vi "eyecat MAX v02.vi"() -> ()   [LabVIEW 2014]
doc: "This VI is an upgrade from the WIN 1_v4 that implements the ageing subrutine"
uses:
  Buttons/String output.ctl
  <vilib>/Utility/miscctls.llb/LVRowAndColumnTypeDef.ctl
  Buttons/Numeric control.ctl
  Buttons/String input.ctl
  Buttons/Numeric indicator.ctl
  Controls Win/Control 3.ctl
  <vilib>/Platform/TimedLoop/XDataNode/nitl_modes.ctl
  <vilib>/Platform/TimedLoop/XDataNode/timing_clust.ctl
  <vilib>/Platform/TimedLoop/XDataNode/wakeup.ctl
  <vilib>/Utility/file.llb/Write To Spreadsheet File (string).vi
  <vilib>/Utility/file.llb/Read From Spreadsheet File (string).vi
  <vilib>/regexp/Match Regular Expression.xnode
  <vilib>/Platform/TimedLoop/XDataNode/XDataNode.xnode
  <vilib>/Platform/TimedLoop/XDataNode/XDNodeRunTimeDep.lvlib
panel:
  out "Furnace temp 2":dbl
  out "output cluster":T2
  out "Full system?":bool
  out "Log interval (seconds)":T1
  in  "Flow rate Age":dbl
  in  "Inlet temp Age":dbl
  out "Stopped?":bool
  in  "Stop Cmd":T1
  out "Connected?":bool
  out "Error":dbl
  out "Iteration Duration":i64
  out "Finished Late? [i-1]":bool
  in  "stop TCP":bool
  in  "SO2 ppm":dbl
  out "Furnace temp 1":dbl
  out "stop 2":bool
  in  "Enum 1":i16=1
  in  "Acknowledge":bool
  out "Test number":u16
  out "Flag1":bool=TRUE
  out "EditPos Subc":T3
  out "Flag 2":bool=TRUE
  in  "Tab Control":T4(tab)
  out "Doors Unlocked":bool
  in  "Temperature Limit (°C)":T1=800.0 min=0.0 max=1200.0 step=1.0
  in  "Log Test Button":bool
  in  "File Name":T5
  in  "File Path":path=path "C:/DATA LOG"
  out "Fail":bool
  out "Pass":bool
  in  "Select Test Type":T6(radio)
  out "Standby":bool
  out "Doors Open":bool
  out "Extractor Fan On":bool
  out "Test In Progress":bool
  out "Cool Down":bool
  out "System Alarm":bool
  in  "Execute Leak Test Button":bool
  in  "Stop Test Button":bool
  in  "Start Test Button":bool
  in  "Advanced settings":bool
  in  "Inlet Temperature (°C)":T1=400.0 min=350.0 max=1000.0 step=1.0
  in  "Inlet LAMBDA Rich":T1=0.9 min=0.85 max=0.96 step=0.001
  in  "Inlet LAMBDA Lean":T1=1.2 min=1.02 max=3.0 step=0.001
  in  "Test Stop temperature (°C)":T1=300.0 min=100.0 max=1000.0 step=1.0
  in  "Test Start Temperature (°C)":T1=125.0 min=0.0 max=500.0 step=1.0
  in  "Furnace Ramp Rate (°C/min)":T1=15.0 min=1.0 max=50.0 step=0.1
  in  "NO:CO Ratio":T1=1.1 min=1.0 max=5.0 step=0.1
  in  "Inlet O2 (%)":T1=0.5 min=0.0 max=14.0 step=0.01
  in  "Inlet LAMBDA":T1=1.0 min=0.6 max=3.0 step=0.001
  out "Space Velocity (h-1)":T7
  out "Vol Flow @ STP (l/min)":T7
  in  "Test Flow Rate(g/s)":T1 min=0.0 max=100.0 step=0.01
  out "Sample Volume (litres)":T7
  in  "Number of Samples":T1=1.0 min=1.0 max=6.0 step=1.0
  in  "Sample Diameter (mm)":T1
  out "CO Theory (%)":T7 format="%#_3g"
  out "CO Theory (%)":T7 format="%#_3g"
  out "HC Theory (%)":T7
  in  "Sample Length (mm)":T1 min=0.0 step=0.5
  in  "NO ppm SW":dbl=500.0 caption="NO (ppm)" min=0.0 max=500.0 step=1.0
  in  "NO ppm Loff":T1 caption="NO ppm"
  in  "Delete sCycle":bool
  in  "Load sCycle":bool
  in  "Save sCycle":bool
  in  "Clear subcycle":bool
  in  "Clear Cycle Pattern":bool
  in  "Save Cycle":bool
  in  "Load Cycle":bool
  in  "Delete Cycle":bool
  out "Test Compiled":bool
  in  "Compile Test Button":bool
  in  "Sub-Cycle List":i32(listbox)=1
  in  "Cycle List":i32(listbox)=2
  out "Total Test Duration (hrs)":T8
  in  "Ageing Gas":enum32{"Radio Selection 1", "Radio Selection 2"}(radio)
  in  "Sub-Cycle Pattern":string[][](table) caption="Subcycle pattern"
  in  "Total Number of Cycles":T1=1.0 min=1.0 max=10000.0 step=1.0
  in  "Cycle Pattern":string[][](table)
  in  "Sub-Cycle Name":T5
  in  "Cycle Name":T5
  out "Heat Exchanger Temperatures (°C)":dynamicdata(graph)
  out "Flow Rate (g/s)":dynamicdata(graph)
  out "Sample Temperatures (°C)":dynamicdata(graph)
  out "System Temperatures (°C)":dynamicdata(graph)
  out "HC Concentration (ppm)":dynamicdata(graph)
  out "Lambda":dynamicdata(graph)
  out "M584L Upstream & Downstream":dynamicdata(graph)
  out "NO Concentration (ppm)":dynamicdata(graph)
  in  "Purge System":bool
  in  "Alarm ack":bool
  in  "Clear log":bool
  out "Table":string[][](table)
  out "Soft Alarm":bool
  out "Hard Alarm":bool
  # "Test Type"
  # "Test Commands"
  # "System Indicators"
  # "Leak Test"
  # "Catalyst Specification"
  # "Lightoff Settings"
  # "Furnace Lightoff Settings"
  # "Sweep Settings"
  # "CO/HC Lightoff Settings"
  # "0.96 < lambda < 0.85"
  # "1.02< lambda < 1.6"
  # "350 < Tinlet < 1000"
  # "NO Lightoff Settings"
  # "Flow Specification"
  # "Cycle Compiled"
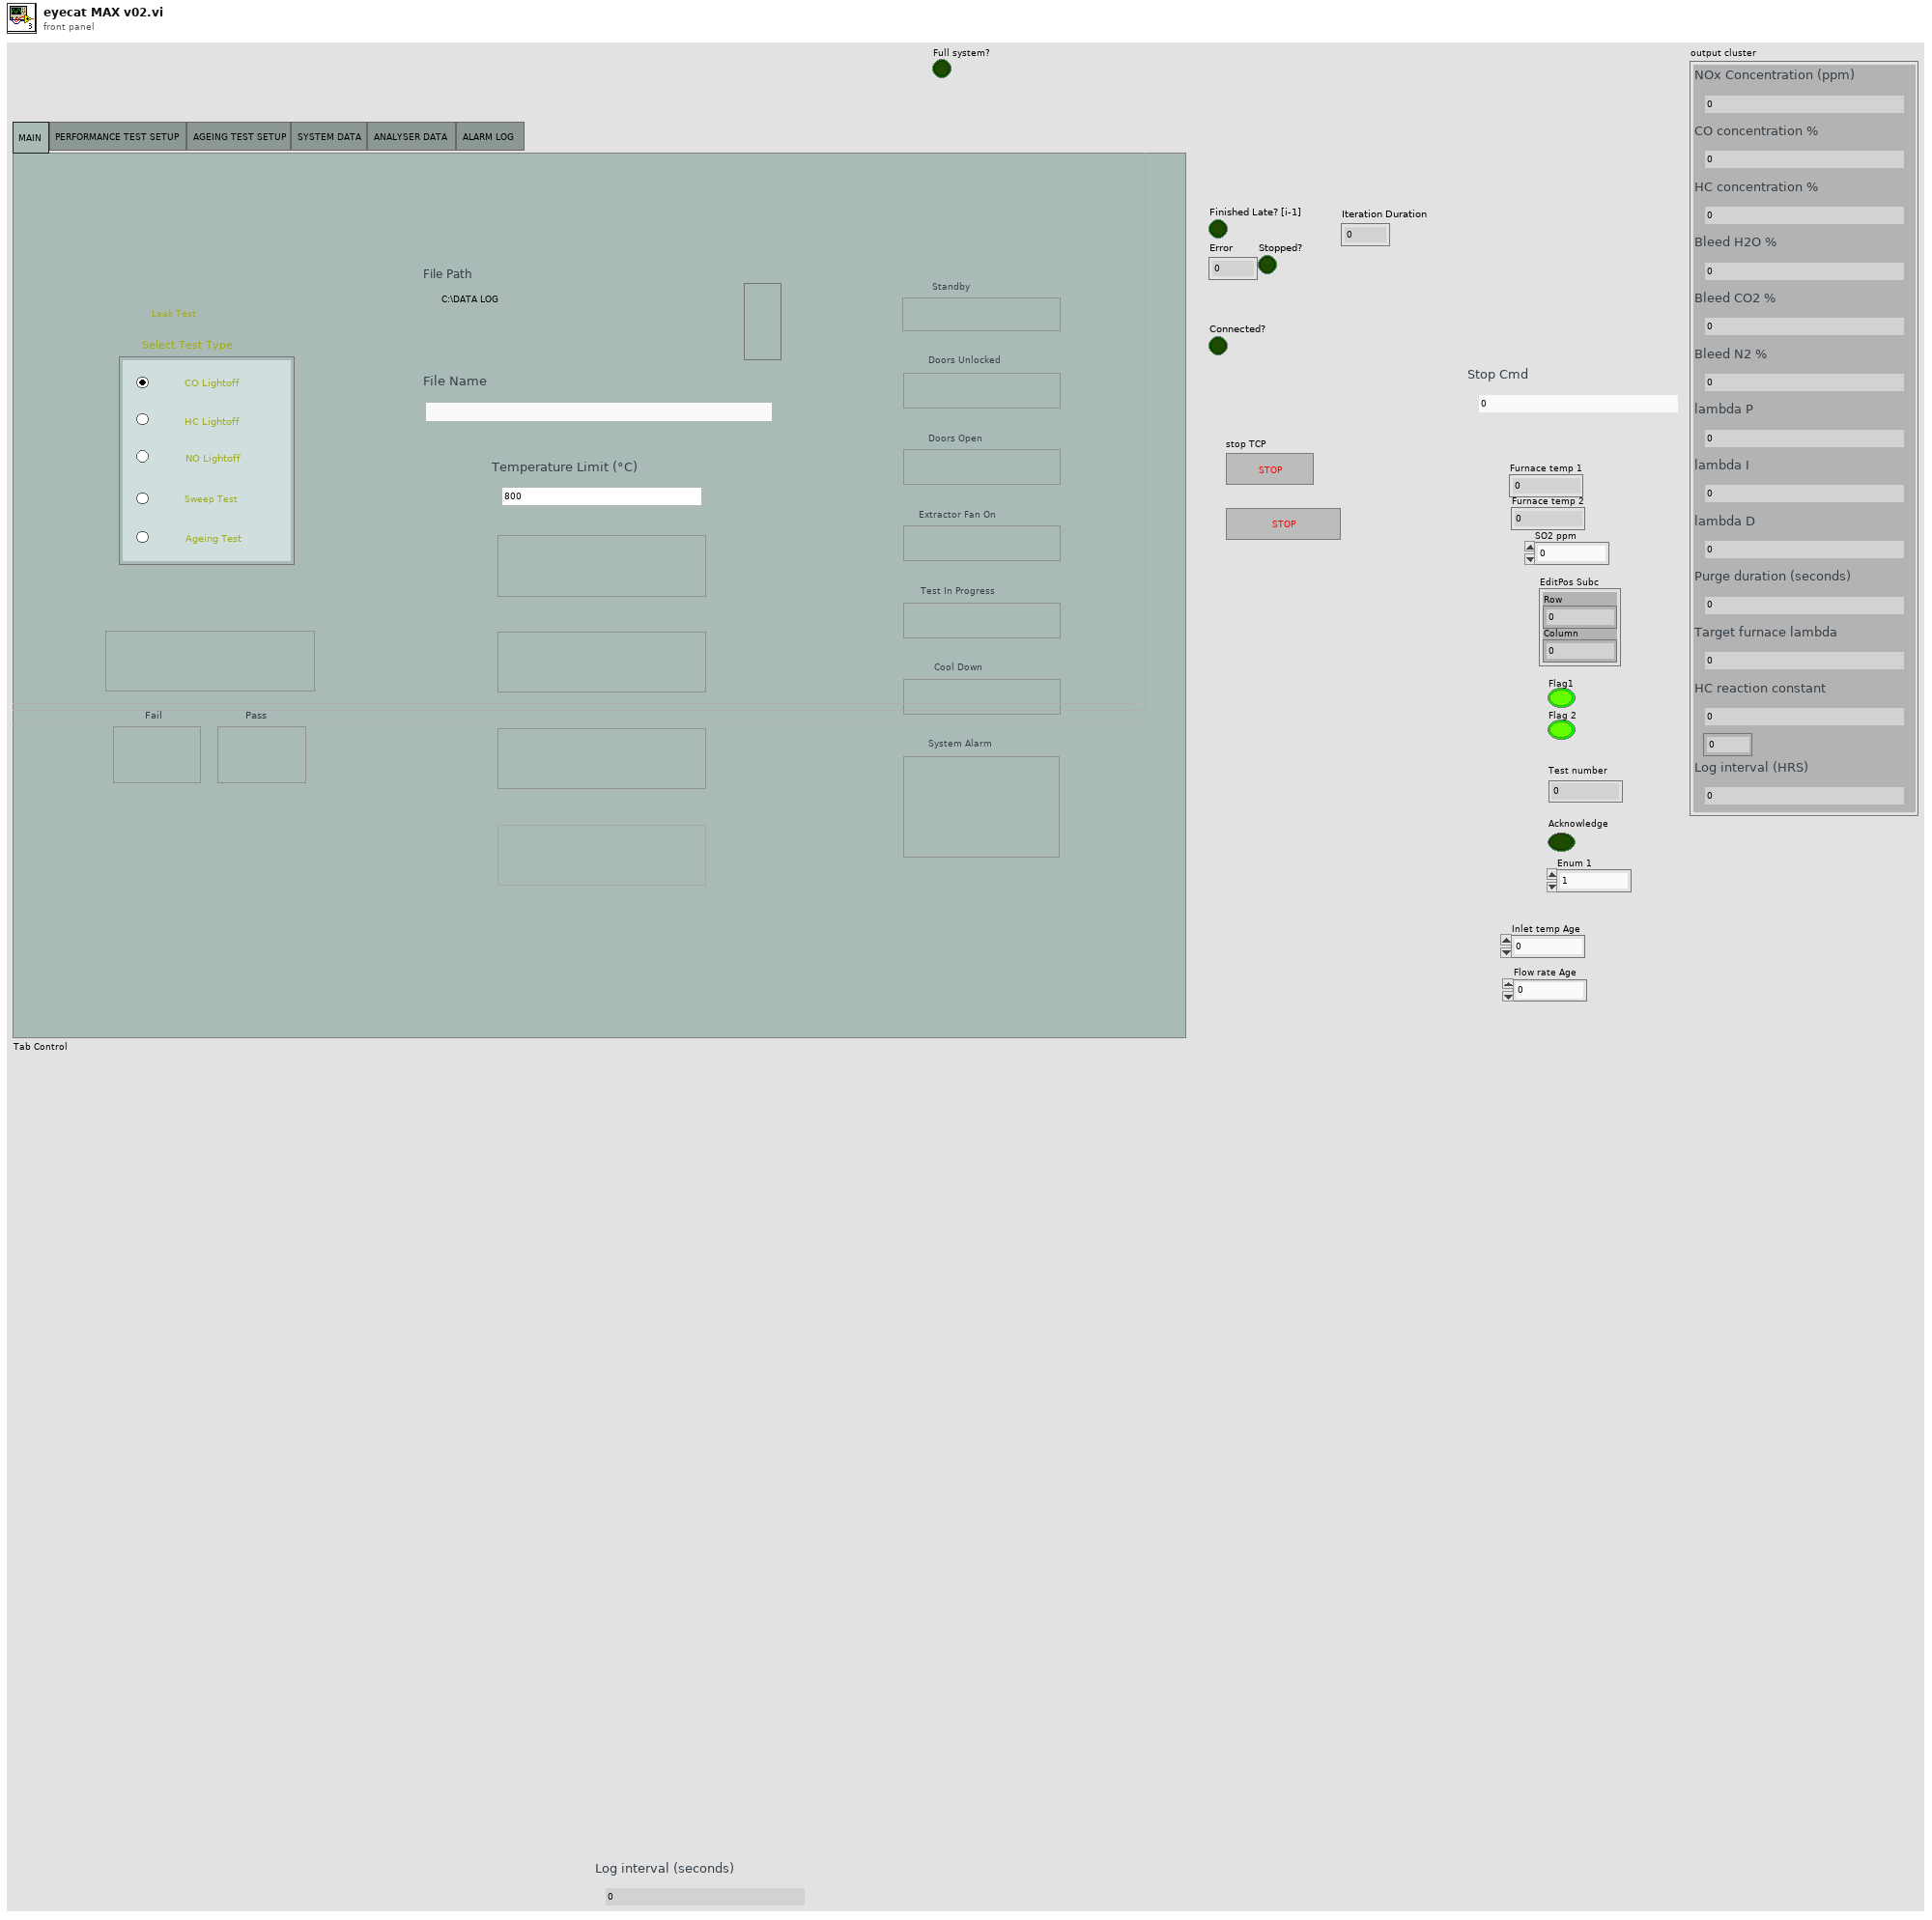
[diagram p1: front panel]
types:
  T1 = typedef "Numeric control.ctl" = dbl
  T2 = cluster{"NOx Concentration (ppm)":T1, "CO concentration %":T1, "HC concentration %":T1, "Bleed H2O %":T1, "Bleed CO2 %":T1, "Bleed N2 %":T1, "lambda P":T1, "lambda I":T1, "lambda D":T1, "Purge duration (seconds)":T1, "Target furnace lambda":T1, "HC reaction constant":T1, i16, "Log interval (HRS)":T1}
  T3 = typedef "LVRowAndColumnTypeDef.ctl" = cluster{"Row":i32, "Column":i32}
  T4 = enum32{"MAIN", "PERFORMANCE TEST SETUP", "AGEING TEST SETUP", "SYSTEM DATA", "ANALYSER DATA", "ALARM LOG"}
  T5 = typedef "String input.ctl" = string
  T6 = enum32{"CO Lightoff", "HC Lightoff", "NO Lightoff", "Sweep Test", "Ageing Test"}
  T7 = typedef "Numeric indicator.ctl" = dbl
  T8 = typedef "String output.ctl" = string
  T9 = typedef "XDNodeRunTimeDep.lvlib/nitl_modes.ctl" = enum32{"No Change", "Process missed periods, maintain original phase", "Discard missed periods, maintain original phase", "Process missed periods, ignore original phase", "Discard missed periods, ignore original phase"}
  T10 = typedef "Control 3.ctl" = enum16{"main", "start test", "save subc", "load subc", "delete subc", "clear table 1", "update list 1", "save cycle", "load cycle", "delete cycle", "clear table 2", "update list 2", "calc HC CO", "Total time calc", "update Cycle pattern ", "load cycle name", "convert to num", "load test array", "check scycle name", "check cycle name", "Multigas connect", "Multigas disconnect"}
  T11 = typedef "XDNodeRunTimeDep.lvlib/timing_clust.ctl" = cluster{"Expected End [f-1]":u64, "Actual End [f-1]":u64, "Finished Late? [f-1]":bool, "Expected End [i-1]":u64, "Actual End [i-1]":u64, "Finished Late? [i-1]":bool, "Expected Start [i]":u64, "Actual Start [i]":u64, "Expected Start [f]":u64, "Actual Start [f]":u64, "Source Name":string, "Structure Name":string, "Period":i64, "Deadline":i64, "Offset":i64, "Start":i64, "Priority":i32, "Timeout":i32, "Mode":T9, "Wakeup Reason":T12, "Error":errorcluster, "Source Type":string, "Secondary Source Type":string, "Global End Time":u64, "Global Start Time":u64, "Frame Duration":u64, "Iteration Duration":u64, "Assigned CPU":i32, "I/O Scan Engine Mode":u32}
  T12 = typedef "XDNodeRunTimeDep.lvlib/wakeup.ctl" = enum32{"Normal", "Aborted", "Asynchronous wakeup", "Timing source error", "Timed loop error", "Timeout"}
  T13 = enum8{"Enabled", "Disabled", "Disabled and Grayed Out"}
  T14 = cluster{"NOx Concentration (ppm)":T1, "CO concentration %":T1, "HC concentration %":T1, "Bleed H2O %":T1, "Bleed CO2 %":T1, "Bleed N2 %":T1, "lambda P":T1, "lambda I":T1, "lambda D":T1, "Purge duration (seconds)":T1, "Target furnace lambda":T1, "HC reaction constant":T1, "Full System?":i16, "Log interval (HRS)":T1}
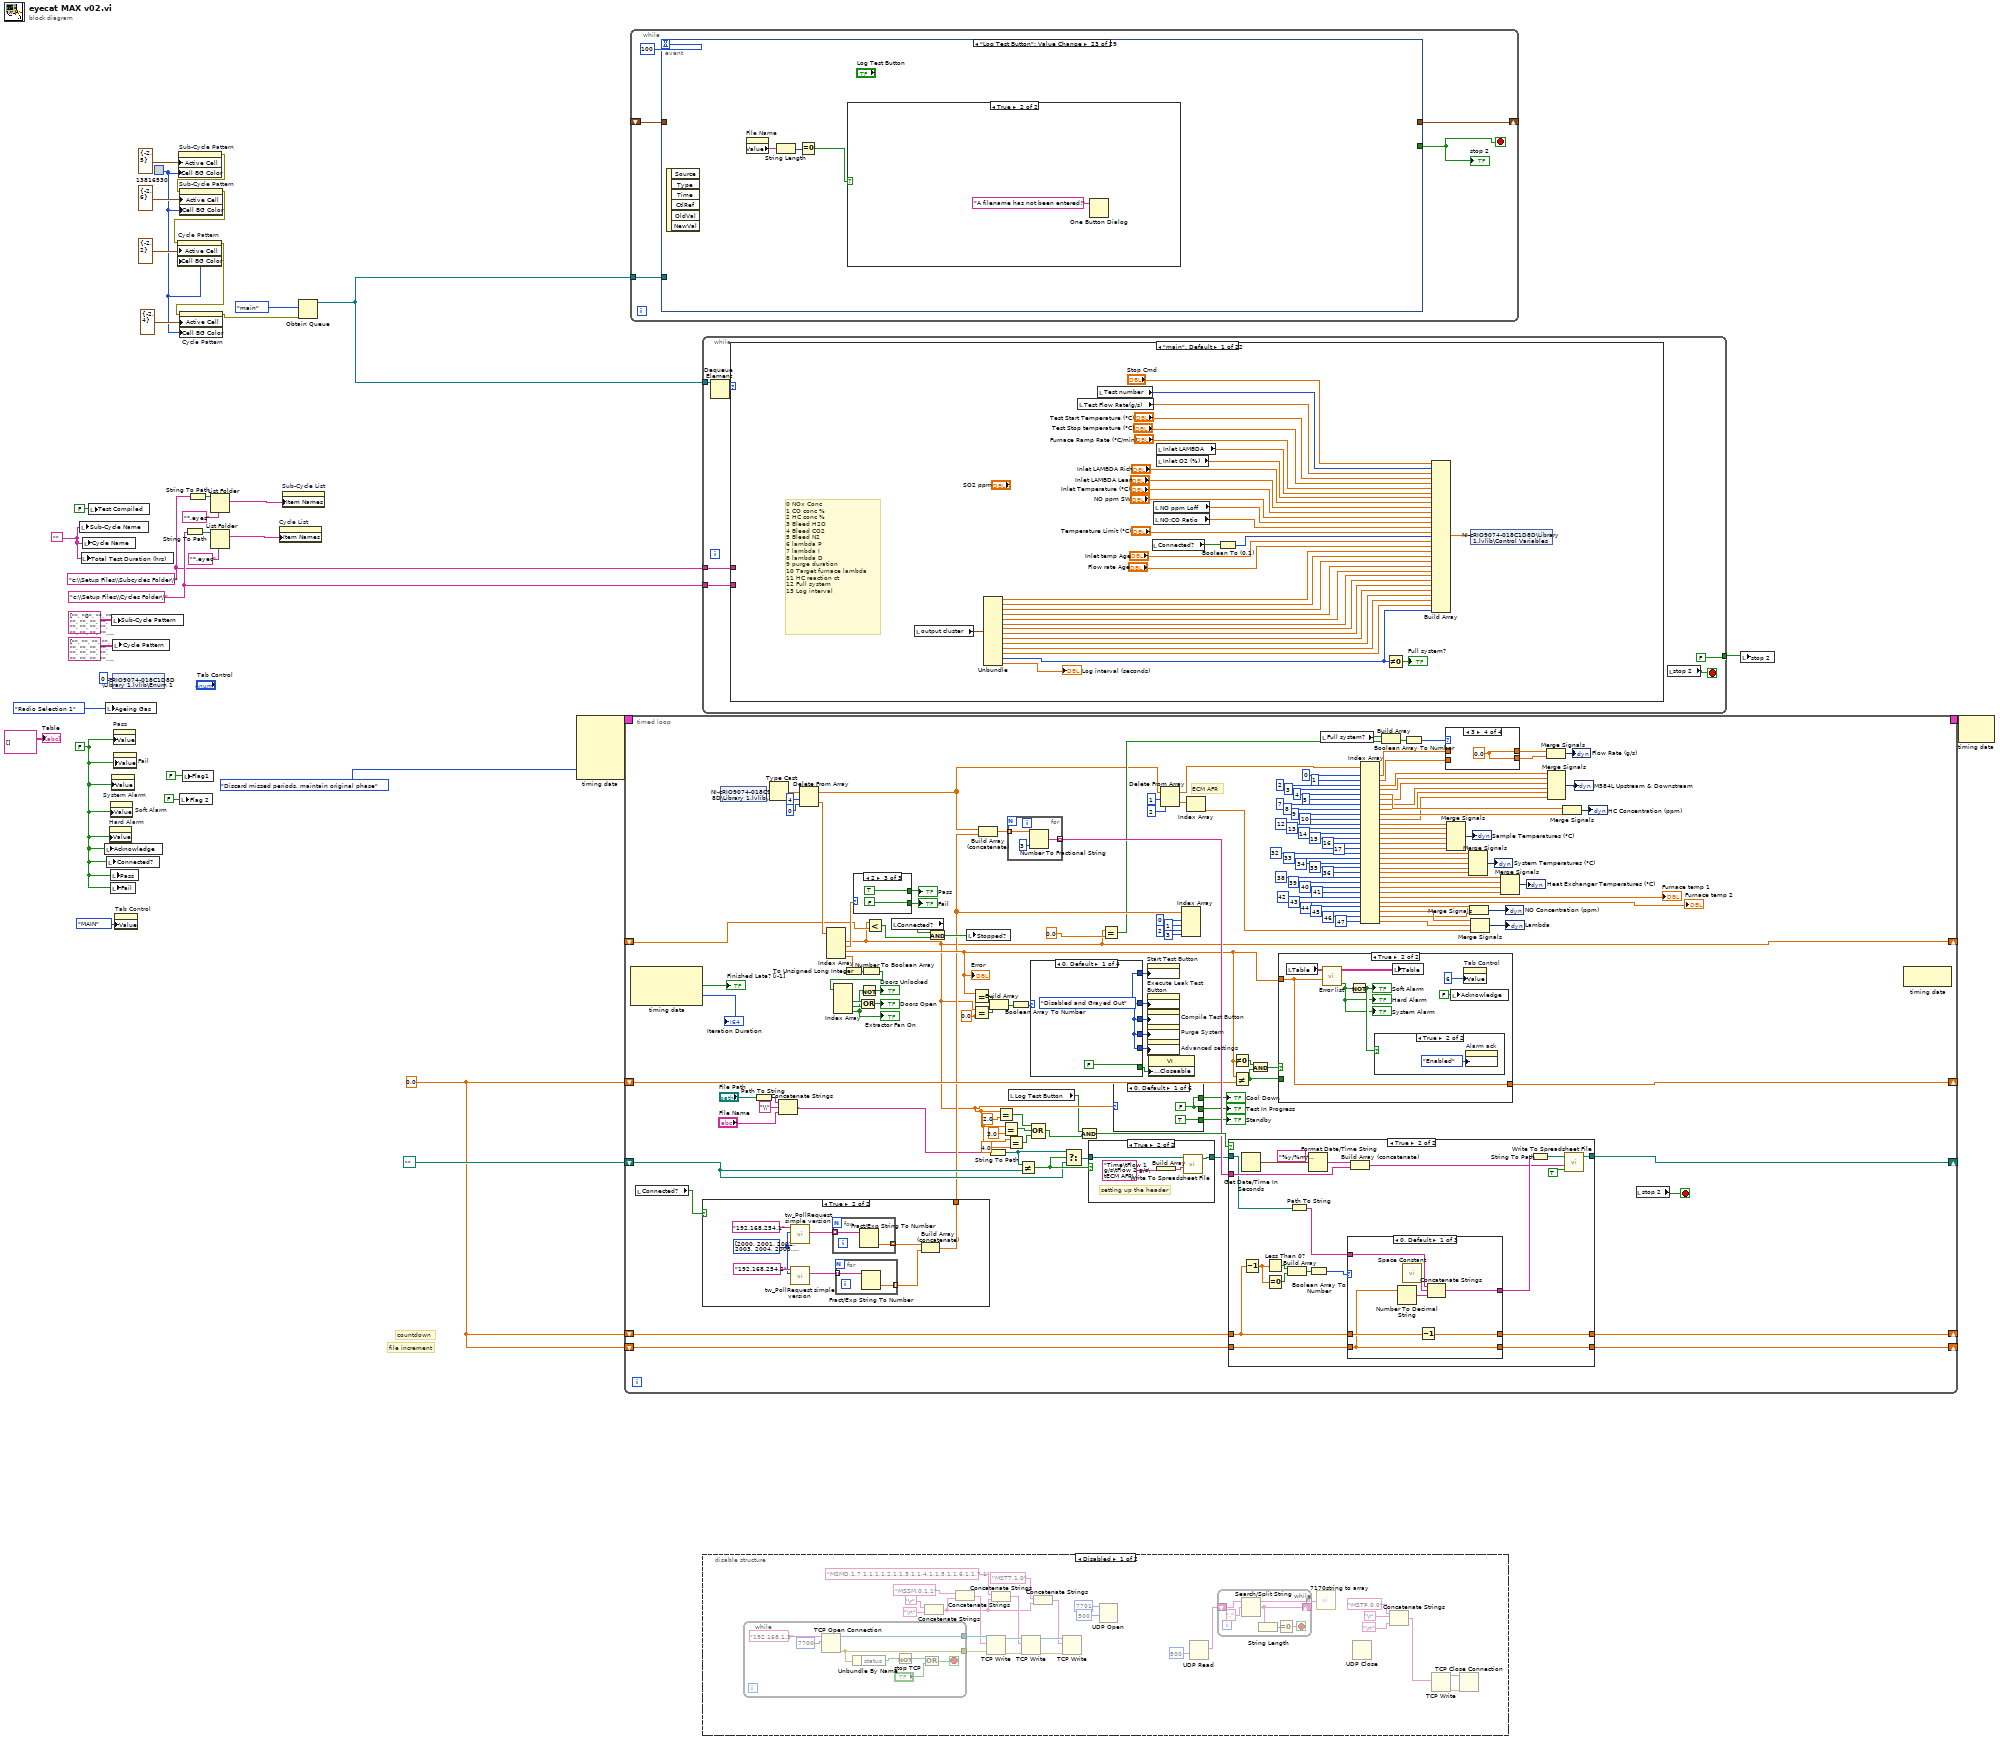
[diagram p0: block diagram]
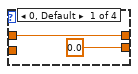
[diagram p3: hidden frame]
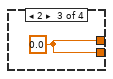
[diagram p5: hidden frame]
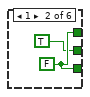
[diagram p6: hidden frame]
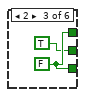
[diagram p7: hidden frame]
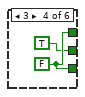
[diagram p8: hidden frame]
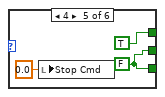
[diagram p9: hidden frame]
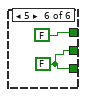
[diagram p10: hidden frame]
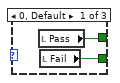
[diagram p11: hidden frame]
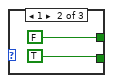
[diagram p12: hidden frame]
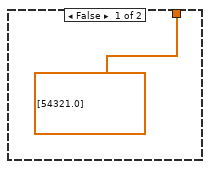
[diagram p13: hidden frame]
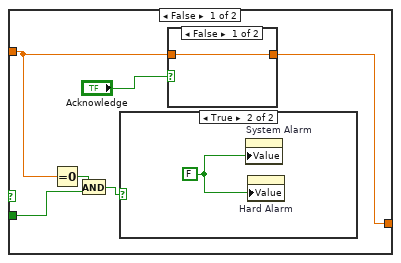
[diagram p14: hidden frame]
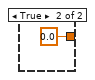
[diagram p15: hidden frame]
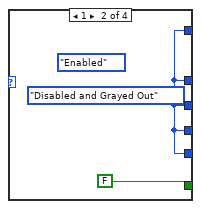
[diagram p18: hidden frame]
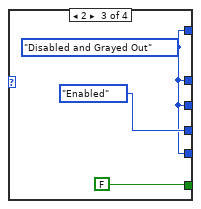
[diagram p19: hidden frame]
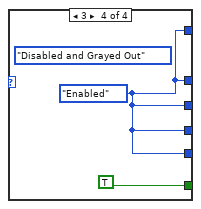
[diagram p20: hidden frame]
diagram:
  w2 = FALSE
  w1 = 0.0 ("y")
  w18 = ""
  w21 = "c:\\Setup Files\\Cycles Folder\\"
  w27 = u32 13816530
  w19 = "c:\\Setup Files\\Subcycles Folder\\"
  # "file increment"
  # "countdown"
  n1 = local write "Sub-Cycle Name"(w18) -> ()
  n2 = local write "Total Test Duration (hrs)"(w18) -> ()
  n3 = local write "Cycle Name"(w18) -> ()
  n4 = local write "Test Compiled"(FALSE ("Cycle Compiled")) -> ()
  n5 = local write "Acknowledge"(w2) -> ()
  n6 = local write "Ageing Gas"(enum32{"Radio Selection 1", "Radio Selection 2"}."Radio Selection 1" ("Ageing Gas")) -> ()
  n7 = local write "Connected?"(w2) -> ()
  n8 = property on="Hard Alarm" class="Bool (strict)"("Value"=w2) -> ()  [unwired: 2 in, 2 out]
  n9 = property on="Soft Alarm" class="Bool (strict)"("Value"=w2) -> ()  [unwired: 2 in, 2 out]
  n10 = local write "Pass"(w2) -> ()
  n11 = local write "Fail"(w2) -> ()
  n12 = local write "Sub-Cycle Pattern"(string[][] [["", "0", "", "", "", "", "", "", "", "", "", "", ""], ["", "", "", "", "", "", "", "", "", "", "", "", ""], ["", "", "", "", "", "", "", "", "", "", "", "", ""], ["", "", "", "", "", "", "", "", "", "", "", "", ""], ["", "", "", "", "", "", "", "", "", "", "", "", ""], ["", "", "", "", "", "", "", "", "", "", "", "", ""], ["", "", "", "", "", "", "", "", "", "", "", "", ""], ["", "", "", "", "", "", "", "", "", "", "", "", ""], ["", "", "", "", "", "", "", "", "", "", "", "", ""], ["", "", "", "", "", "", "", "", "", "", "", "", ""], ["", "", "", "", "", "", "", "", "", "", "", "", ""], ["", "", "", "", "", "", "", "", "", "", "", "", ""], ["", "", "", "", "", "", "", "", "", "", "", "", ""], ["", "", "", "", "", "", "", "", "", "", "", "", ""], ["", "", "", "", "", "", "", "", "", "", "", "", ""], ["", "", "", "", "", "", "", "", "", "", "", "", ""], ["", "", "", "", "", "", "", "", "", "", "", "", ""], ["", "", "", "", "", "", "", "", "", "", "", "", ""], ["", "", "", "", "", "", "", "", "", "", "", "", ""], ["", "", "", "", "", "", "", "", "", "", "", "", ""], ["", "", "", "", "", "", "", "", "", "", "", "", ""], ["", "", "", "", "", "", "", "", "", "", "", "", ""], ["", "", "", "", "", "", "", "", "", "", "", "", ""], ["", "", "", "", "", "", "", "", "", "", "", "", ""], ["", "", "", "", "", "", "", "", "", "", "", "", ""], ["", "", "", "", "", "", "", "", "", "", "", "", ""], ["", "", "", "", "", "", "", "", "", "", "", "", ""], ["", "", "", "", "", "", "", "", "", "", "", "", ""], ["", "", "", "", "", "", "", "", "", "", "", "", ""], ["", "", "", "", "", "", "", "", "", "", "", "", ""], ["", "", "", "", "", "", "", "", "", "", "", "", ""]]) -> ()
  n13 = property on="System Alarm" class="Bool (strict)"("Value"=w2) -> ()  [unwired: 2 in, 2 out]
  n14 = local write "Cycle Pattern"(string[][] [["", "", "", "", ""], ["", "", "", "", ""], ["", "", "", "", ""], ["", "", "", "", ""], ["", "", "", "", ""], ["", "", "", "", ""], ["", "", "", "", ""], ["", "", "", "", ""], ["", "", "", "", ""], ["", "", "", "", ""], ["", "", "", "", ""], ["", "", "", "", ""], ["", "", "", "", ""], ["", "", "", "", ""], ["", "", "", "", ""], ["", "", "", "", ""], ["", "", "", "", ""], ["", "", "", "", ""], ["", "", "", "", ""], ["", "", "", "", ""], ["", "", "", "", ""], ["", "", "", "", ""], ["", "", "", "", ""], ["", "", "", "", ""], ["", "", "", "", ""], ["", "", "", "", ""], ["", "", "", "", ""], ["", "", "", "", ""], ["", "", "", "", ""], ["", "", "", "", ""], ["", "", "", "", ""]]) -> ()
  n15 = shared-variable "NI-cRIO9074-018C1D8D\\Library 1.lvlib\\Enum 1"(u16 0 ("Enum 1")) -> ()  [unwired: 1 in, 1 out]
  n16 = property on="Pass" class="Bool (strict)"("Value"=w2) -> ()  [unwired: 2 in, 2 out]
  n17 = property on="Fail" class="Bool (strict)"("Value"=w2) -> ()  [unwired: 2 in, 2 out]
  n18 = property on="Tab Control" class="TabCtl (strict)"("Value"=T4."MAIN" ("Tab Control")) -> ()  [unwired: 2 in, 2 out]
  n19 = property on="Sub-Cycle Pattern" class="Tbl (strict)"("Active Cell"=T3 {"Row"=-2, "Column"=5} ("Active Cell:Active Cell"), "Cell BG Color"=w27) -> (error out=w32:errorcluster)  [unwired: 2 in, 1 out]
  n20 = property on="Sub-Cycle Pattern" class="Tbl (strict)"(error in=w32, "Active Cell"=T3 {"Row"=-2, "Column"=6} ("Active Cell:Active Cell"), "Cell BG Color"=w27) -> (error out=w31:errorcluster)  [unwired: 1 in, 1 out]
  n21 = property on="Cycle Pattern" class="Tbl (strict)"(error in=w31, "Active Cell"=T3 {"Row"=-2, "Column"=2} ("Active Cell:Active Cell"), "Cell BG Color"=w27) -> (error out=w29:errorcluster)  [unwired: 1 in, 1 out]
  n22 = property on="Cycle Pattern" class="Tbl (strict)"(error in=w29, "Active Cell"=T3 {"Row"=-2, "Column"=4} ("Active Cell:Active Cell"), "Cell BG Color"=w27) -> (error out=w26:errorcluster)  [unwired: 1 in, 1 out]
  n23 = local write "Flag 2"(FALSE) -> ()
  n24 = local write "Flag1"(FALSE) -> ()
  n25 = String To Path(string=w21) -> (path=w22:path)
  n26 = String To Path(string=w19) -> (path=w24:path)
  n27 = List Folder(path=w22, pattern="*.eyec") -> (filenames=w23:string[])  [unwired: 2 in, 3 out]
  n28 = List Folder(path=w24, pattern="*.eyes") -> (filenames=w25:string[])  [unwired: 2 in, 3 out]
  n29 = property on="Cycle List" class="LstBox (strict)"("Item Names"=w23) -> ()  [unwired: 2 in, 2 out]
  n30 = property on="Sub-Cycle List" class="LstBox (strict)"("Item Names"=w25) -> ()  [unwired: 2 in, 2 out]
  n31 = Obtain Queue(element data type=Control_3."main" ("Enum"), error in (no error)=w26) -> (queue out=w35:refnum<queue>)  [unwired: 3 in, 2 out]
  n32 = node-c288(nitl_modes."Discard missed periods, maintain original phase" ("Mode")) -> (w7:T11)  [unwired: 4 in]
  n33 = timed-loop {
    timing: w7 -> [_]
    timing-out: [_] -> w6
    shift-right: [w166] -> _
    shift-left: path "" -> [w168]
    shift-right: [w120] -> _
    shift-left: w1 -> [w167]
    shift-right: [w40] -> _
    shift-left: _ -> [w131]
    shift-right: [w110] -> _
    shift-left: w1 -> [w113]
    shift-right: [w111] -> _
    shift-left: w1 -> [w112]
    stop <- w165 stop-if-true
    w148 = 0.0 ("y")
    # "ECM AFR"
    n34 = node-c288() -> (→"Finished Late? [i-1]":bool, →"Iteration Duration":i64)  [unwired: 1 in, 1 out]
    n35 = local read "Connected?"() -> (w154:bool)
    n36 = case shown="True" w154 {
      tunnel: [dbl[] [54321.0] ("Output") w222] -> w109
      frame False {
      }
      frame True {
        w225 = i32[] [2000, 2001, 2002, 2003, 2004, 2005, 2006, 2007, 2008, 2009, 2010, 2011, 2012, 2013, 2014] ("EVID list")
        n37 = call "tw_PollRequest simple version.vi"("EVID list"=w225, "IP_ADD [127.0.0.1]"="192.168.254.1") -> ("values out"=w228:string[])  [unwired: 7 in, 2 out]
        n38 = call "tw_PollRequest simple version.vi"("EVID list"=w225, "IP_ADD [127.0.0.1]"="192.168.254.2") -> ("values out"=w227:string[])  [unwired: 7 in, 2 out]
        n39 = for {
          tunnel: [w233] -> w223 mode=indexing
          tunnel: w228 -> [w232] mode=indexing
          n40 = Fract/Exp String To Number(string=w232) -> (number=w233:dbl)  [unwired: 3 in, 1 out]
        }
        n41 = for {
          tunnel: [w231] -> w224 mode=indexing
          tunnel: w227 -> [w230] mode=indexing
          n42 = Fract/Exp String To Number(string=w230) -> (number=w231:dbl)  [unwired: 3 in, 1 out]
        }
        n43 = Build Array (concatenate)(w223, w224) -> (w222:dbl[])
      }
    }
    n44 = shared-variable "NI-cRIO9074-018C1D8D\\Library 1.lvlib\\DATA"() -> (w164:dbl[])  [unwired: 1 in, 1 out]
    n45 = Path To String(path="File Path") -> (string=w124:string)
    n46 = Type Cast(type=w164, x=w164) -> (*(type *) &x=w176:dbl[])
    n47 = Concatenate Strings(w124, "\\" ("string"), "File Name") -> (w37:string)
    n48 = Delete From Array(array=w176, length=4, index=0) -> (deleted portion=w173:dbl[], array with subset deleted=w50:dbl[])
    n49 = Index Array(array=w173) -> (element #1=w40:dbl, element #2=w137:dbl, element #3=w138:dbl, element #4=w130:dbl)  [unwired: 4 in]
    "Error" <- w138
    n50 = To Unsigned Long Integer(number=w130) -> (unsigned 32bit integer=w129:u32)
    n51 = case shown="2" w137 {
      tunnel: [w215 TRUE FALSE] -> w136
      tunnel: [w216 FALSE TRUE] -> w135
      frame 0, Default {
        n52 = local read "Pass"() -> (w216:bool)
        n53 = local read "Fail"() -> (w215:bool)
      }
      frame 1 {
      }
      frame 2 {
      }
    }
    "Pass" <- w135
    "Fail" <- w136
    n54 = Number To Boolean Array(number=w129) -> (Boolean array=w153:bool[])
    n55 = Index Array(array=w153) -> (element #2=w151:bool, element #3=w150:bool, element #4=w126:bool)  [unwired: 4 in, 1 out]
    "Extractor Fan On" <- w126
    n56 = Or(x=w151, y=w150) -> (x .or. y?=→"Doors Open":bool)
    n57 = Not(x=w126) -> (.not. x?=→"Doors Unlocked":bool)
    n58 = Less?(x=w40, y=w131) -> (x < y?=w128:bool)
    n59 = local read "Connected?"() -> (w127:bool)
    n60 = And(x=w127, y=w128) -> (x .and. y?=w119:bool)
    n61 = local write "Stopped?"(w119) -> ()
    n62 = Equal?(x=w138, y=w148) -> (x = y?=w146:bool)
    n63 = Equal?(x=w40, y=w148) -> (x = y?=w145:bool)
    n64 = Build Array (concatenate)(w50, w109) -> (w169:dbl[])
    n65 = String To Path(string=w37) -> (path=w121:path)
    n66 = Build Array(w146, w145) -> (w144:bool[])
    n67 = Equal?(x=w40, y=2.0) -> (x = y?=w52:bool)
    n68 = Equal?(x=w40, y=3.0) -> (x = y?=w43:bool)
    n69 = Equal?(x=w40, y=4.0) -> (x = y?=w41:bool)
    n70 = for {
      tunnel: w169 -> [w266] mode=indexing
      tunnel: [w265] -> w180 mode=indexing
      n71 = Number To Fractional String(number=w266, precision (6)=i16 3) -> (F-format string=w265:string)  [unwired: 2 in]
    }
    n72 = local read "Log Test Button"() -> (w38:bool)
    n73 = Boolean Array To Number(Boolean array=w144) -> (number=w143:u32)
    n74 = Not Equal?(x=w121, y=w168) -> (x != y?=w178:bool)
    n75 = case shown="0, Default" w143 {
      tunnel: [w252 w254 w256 w259] -> w147
      tunnel: [w252 w254 w256 w259] -> w142
      tunnel: [w252 w254 w256 w259] -> w141
      tunnel: [w252 w254 T13."Enabled" ("Disabled") w259] -> w140
      tunnel: [w252 w254 w256 w259] -> w139
      tunnel: [FALSE FALSE FALSE TRUE] -> w118
      frame 0, Default {
        w252 = T13."Disabled and Grayed Out" ("Disabled")
      }
      frame 1 {
        (unwired) T13."Enabled" ("Disabled")
        w254 = T13."Disabled and Grayed Out" ("Disabled")
      }
      frame 2 {
        w256 = T13."Disabled and Grayed Out" ("Disabled")
      }
      frame 3 {
        w259 = T13."Enabled" ("Disabled")
        (unwired) T13."Disabled and Grayed Out" ("Disabled")
      }
    }
    n76 = Compound Arithmetic op=OR(w52, w43, w41) -> (w51:bool)
    n77 = Select(t=w121, s=w178, f=w168) -> (s? t:f=w179:path)
    n78 = And(x=w38, y=w51) -> (x .and. y?=w195:bool)
    n79 = case shown="True" w178 {
      tunnel: w179 -> [w260 w264]
      tunnel: [w260 w263] -> w177
      frame False {
      }
      frame True {
        # "setting up the header"
        n80 = Build Array("Time\tFlow 1 g/s\tFlow 2 g/s\tECM AFR\tCO2 U %\tCO U %\tHC U ppm\tO2 U %\tNO U ppm\tCO2 D %\tCO D %\tHC D ppm\tO2 D %\tNO D ppm\tTC1X\tTC2A\tTCY\tTC4B\tTC5\tTC6\tTC7\tTC8\tTC9\tTC10\tTC11\tTC12\tTC13\tTC14\tTC15\tTC16\tTC17\tTC18\tTC19\tTC20\tTC Vent 1\tTC Vent 2\tTC Fan B1\tTC Fan B2\tTC Cab\tTC Ex A\tTC Ex B\tTC Ex C\tTC Ex D\tTC Furn 1\tTC Furn 2\tNOX 1 ppm\tNLambda 1\tNOX 2 ppm\tNLambda 2\tEGO 1\tEGO 2\tEGO 3\tEGO 4\tCO2 U %\tCO U %\tHC U ppm\tO2 U %\tNO U ppm\tCO2 D %\tCO D %\tHC D ppm\tO2 D %\tNO D ppm\r\n" ("Heading string 2")) -> (w262:string[])
        n81 = call-poly <vilib>:"Write To Spreadsheet File.vi"("1D data"=w262, "file path (dialog if empty)"=w264) -> ("new file path (Not A Path if cancelled)"=w263:path)  [unwired: 6 in]
      }
    }
    n82 = Equal?(x=w40, y=0.0) -> (x = y?=w106:bool)
    n83 = case shown="0, Default" w40 {
      tunnel: [w202 w205 w207 w209 TRUE FALSE] -> w134
      tunnel: [w202 TRUE TRUE TRUE w211 w213] -> w133
      tunnel: [TRUE w205 w207 w209 w211 w213] -> w132
      frame 0, Default {
        w202 = FALSE
      }
      frame 1 {
        w205 = FALSE
      }
      frame 2 {
        w207 = FALSE
      }
      frame 3 {
        w209 = FALSE
      }
      frame 4 {
        w211 = FALSE
        n84 = local write "Stop Cmd"(T1 0.0 ("Stop Cmd")) -> ()
      }
      frame 5 {
        w213 = FALSE
      }
    }
    "Cool Down" <- w134
    "Test In Progress" <- w133
    "Standby" <- w132
    n85 = property on="Start Test Button" class="Bool"("DisabledEnum"=w147) -> ()  [unwired: 2 in, 2 out]
    n86 = property on="Execute Leak Test Button" class="Bool"("DisabledEnum"=w142) -> ()  [unwired: 2 in, 2 out]
    n87 = property on="Compile Test Button" class="Bool"("DisabledEnum"=w141) -> ()  [unwired: 2 in, 2 out]
    n88 = property on="Purge System" class="Bool"("DisabledEnum"=w140) -> ()  [unwired: 2 in, 2 out]
    n89 = property on="Advanced settings" class="Bool"("DisabledEnum"=w139) -> ()  [unwired: 2 in, 2 out]
    n90 = property class="VI"("Front Panel.Closeable"=w118) -> ()  [unwired: 2 in, 2 out]
    n91 = Delete From Array(array=w50, length=1, index=2) -> (deleted portion=w47:dbl[], array with subset deleted=w45:dbl[])
    n92 = Index Array(array=w109, index #1=0 ("index"), index #2=1 ("index"), index #3=2 ("index"), index #4=3 ("index")) -> ()  [unwired: 4 out]
    n93 = Index Array(array=w47) -> (element=w46:dbl)  [unwired: 1 in]
    n94 = case shown="True" w195 {
      tunnel: w177 -> [w270 w278]
      tunnel: [w270 w290] -> w166
      tunnel: w180 -> [_ w286]
      tunnel: w113 -> [_ w279]
      tunnel: w112 -> [w269 w274]
      tunnel: [w269 w276] -> w111
      tunnel: [w268 w275] -> w110
      frame False {
        n95 = local read "Log interval (seconds)"() -> (w268:T1)
      }
      frame True {
        n96 = Get Date/Time In Seconds() -> (seconds since 1Jan1904=w287:timestamp)
        n97 = Decrement(x=w279) -> (x-1=w280:T1)
        n98 = Less Than 0?(x=w280) -> (x < 0?=w281:bool)
        n99 = Equal To 0?(x=w280) -> (x = 0?=w282:bool)
        n100 = Build Array(w281, w282) -> (w283:bool[])
        n101 = Path To String(path=w278) -> (string=w273:string)
        n102 = Format Date/Time String(time format string (%c)="%y/%m/%d %H:%M:%S", seconds (now)=w287) -> (date/time string=w288:string)  [unwired: 1 in]
        n103 = Boolean Array To Number(Boolean array=w283) -> (number=w284:u32)
        n104 = case shown="0, Default" w284 {
          tunnel: w279 -> [w297 w298 _]
          tunnel: [w296 w298 w301] -> w275
          tunnel: w273 -> [w295 w300 w304]
          tunnel: [w292 w300 w302] -> w277
          tunnel: [w291 w299 w303] -> w276
          tunnel: w274 -> [w291 w299 w307]
          frame 0, Default {
            n105 = Number To Decimal String(number=w291) -> (decimal integer string=w293:string)  [unwired: 1 in]
            n106 = call <vilib>:"Space Constant.vi"() -> ("String"=w294:string)
            n107 = Decrement(x=w297) -> (x-1=w296:T1)
            n108 = Concatenate Strings(w295, w294, w293) -> (w292:string)
          }
          frame 1 {
          }
          frame 2 {
            n109 = local read "Log interval (seconds)"() -> (w301:T1)
            n110 = Increment(x=w307) -> (x+1=w303:dbl)
            n111 = Number To Decimal String(number=w303) -> (decimal integer string=w305:string)  [unwired: 1 in]
            n112 = call <vilib>:"Space Constant.vi"() -> ("String"=w306:string)
            n113 = Concatenate Strings(w304, w306, w305) -> (w302:string)
          }
        }
        n114 = Build Array (concatenate)(w288, w286) -> (w272:string[])
        n115 = String To Path(string=w277) -> (path=w271:path)
        n116 = call-poly <vilib>:"Write To Spreadsheet File.vi"("append to file? (new file:F)"=TRUE, "1D data"=w272, "file path (dialog if empty)"=w271) -> ("new file path (Not A Path if cancelled)"=w290:path)  [unwired: 5 in]
      }
    }
    n117 = Not Equal To 0?(x=w138) -> (x != 0?=w171:bool)
    n118 = Not Equal?(x=w138, y=w167) -> (x != y?=w170:bool)
    n119 = And(x=w171, y=w170) -> (x .and. y?=w172:bool)
    n120 = case shown="True" w172 {
      tunnel: w138 -> [w235 w246]
      tunnel: w170 -> [w238 _]
      tunnel: [w234 w246] -> w120
      frame False {
        n121 = Equal To 0?(x=w235) -> (x = 0?=w239:bool)
        n122 = And(x=w239, y=w238) -> (x .and. y?=w237:bool)
        n123 = case shown="True" w237 {
          frame False {
          }
          frame True {
            w242 = FALSE ("Ack hard alarm!")
            n124 = property on="System Alarm" class="Bool (strict)"("Value"=w242) -> ()  [unwired: 2 in, 2 out]
            n125 = property on="Hard Alarm" class="Bool (strict)"("Value"=w242) -> ()  [unwired: 2 in, 2 out]
          }
        }
        n126 = case shown="False" "Acknowledge" {
          tunnel: [w240 0.0 ("Numeric")] -> w234
          tunnel: w235 -> [w240 _]
          frame False {
          }
          frame True {
          }
        }
      }
      frame True {
        n127 = local read "Table"() -> (w249:string[][])
        n128 = call "Error list.vi"("Error code"=w246, "Error array in"=w249) -> ("Hard alarm?"=w243:bool, "Error array out"=w248:string[][])  [unwired: 8 in]
        "Hard Alarm" <- w243
        "System Alarm" <- w243
        n129 = Not(x=w243) -> (.not. x?=w244:bool)
        "Soft Alarm" <- w244
        n130 = case shown="True" w244 {
          frame False {
          }
          frame True {
            n131 = property on="Alarm ack" class="Bool"("DisabledEnum"=T13."Enabled" ("Disabled")) -> ()  [unwired: 2 in, 2 out]
          }
        }
        n132 = local write "Table"(w248) -> ()
        n133 = local write "Acknowledge"(FALSE ("Acknowledge")) -> ()
        n134 = property on="Tab Control" class="TabCtl (strict)"("Value"=6) -> ()  [unwired: 2 in, 2 out]
      }
    }
    n135 = local read "Full system?"() -> (w107:bool)
    n136 = Index Array(array=w45, index #1=0 ("index"), index #2=1 ("index"), index #3=2 ("index"), index #4=3 ("index"), index #5=4 ("index"), index #6=5 ("index"), index #7=7 ("index"), index #8=8 ("index"), index #9=9 ("index"), index #10=10 ("index"), index #11=12 ("index"), index #12=13 ("index"), index #13=14 ("index"), index #14=15 ("index"), index #15=16 ("index"), index #16=17 ("index"), index #17=32 ("index"), index #18=33 ("index"), index #19=34 ("index"), index #20=35 ("index"), index #21=36 ("index"), index #22=38 ("index"), index #23=39 ("index"), index #24=40 ("index"), index #25=41 ("index"), index #26=42 ("index"), index #27=43 ("index"), index #28=44 ("index"), index #29=45 ("index"), index #30=46 ("index"), index #31=47 ("index")) -> (element #1=w104:dbl, element #2=w103:dbl, element #3=w100:dbl, element #4=w98:dbl, element #5=w99:dbl, element #6=w97:dbl, element #7=w96:dbl, element #8=w95:dbl, element #9=w94:dbl, element #10=w93:dbl, element #11=w88:dbl, element #12=w87:dbl, element #13=w86:dbl, element #14=w85:dbl, element #15=w84:dbl, element #16=w83:dbl, element #17=w77:dbl, element #18=w76:dbl, element #19=w75:dbl, element #20=w74:dbl, element #21=w73:dbl, element #22=w68:dbl, element #23=w67:dbl, element #24=w66:dbl, element #25=w65:dbl, element #26=→"Furnace temp 1":dbl, element #27=→"Furnace temp 2":dbl, element #28=w58:dbl, element #29=w57:dbl, element #30=w54:dbl, element #31=w53:dbl)
    n137 = Build Array(w107, w106) -> (w108:bool[])
    n138 = Boolean Array To Number(Boolean array=w108) -> (number=w105:u32)
    n139 = case shown="3" w105 {
      tunnel: w104 -> [w197 w199 _ _]
      tunnel: w103 -> [_ w198 _ _]
      tunnel: [w197 w199 w200 w201] -> w102
      tunnel: [0.0 ("y") w198 w200 w201] -> w101
      frame 0, Default {
      }
      frame 1 {
      }
      frame 2 {
        w200 = 0.0 ("y")
      }
      frame 3 {
        w201 = 0.0 ("y")
      }
    }
    n140 = Merge Signals(w88, w87, w86, w85, w84, w83) -> (→"Sample Temperatures (°C)":dynamicdata)
    n141 = Merge Signals(w77, w76, w75, w74, w73) -> (→"System Temperatures (°C)":dynamicdata)
    n142 = Merge Signals(w58, w54) -> (→"NO Concentration (ppm)":dynamicdata)
    n143 = Merge Signals(w57, w53, w46) -> (→"Lambda":dynamicdata)
    n144 = Merge Signals(w68, w67, w66, w65) -> (→"Heat Exchanger Temperatures (°C)":dynamicdata)
    n145 = Merge Signals(w102, w101) -> (→"Flow Rate (g/s)":dynamicdata)
    n146 = Merge Signals(w100, w98, w97, w96, w95, w93) -> (→"M584L Upstream & Downstream":dynamicdata)
    n147 = Merge Signals(w99, w94) -> (→"HC Concentration (ppm)":dynamicdata)
    n148 = local read "stop 2"() -> (w165:bool)
    n149 = node-c288() -> ()  [unwired: 1 in, 1 out]
  }
  n150 = while {
    tunnel: w35 -> [w316]
    shift-right: [w314] -> _
    shift-left: _ -> [w313]
    stop <- w312 stop-if-true
    n151 = event shown="[22] \"Log Test Button\": Value Change" {
      selector: _ -> [_ _ _ _ _ _ _ _ _ _ _ _ _ _ _ _ _ _ _ _ _ _ _ _ _ _ _ _ _]
      dyn-events: _ -> [_ _ _ _ _ _ _ _ _ _ _ _ _ _ _ _ _ _ _ _ _ _ _ _ _ _ _ _ _]
      timeout: 100 -> [_ _ _ _ _ _ _ _ _ _ _ _ _ _ _ _ _ _ _ _ _ _ _ _ _ _ _ _ _]
      tunnel: w316 -> [w319 w321 _ w330 w338 w345 w352 w363 w367 w378 w383 w386 w391 w413 w421 w422 _ _ _ _ w466 w478 _ w512 w530 _ w544 _ _]
      tunnel: [w317 w320 _ w331 w337 w344 w351 w362 w365 w373 w380 w385 w389 w410 _ _ _ _ _ _ _ _ _ _ _ _ _ _ _] -> w314
      tunnel: w313 -> [w317 w320 _ w331 w337 w344 w350 w362 w365 w373 w380 w385 w389 w410 _ _ _ _ _ _ _ _ _ _ _ _ _ _ _]
      tunnel: [_ _ w323 _ _ _ _ _ _ _ _ _ _ _ _ _ _ _ _ _ _ _ _ _ _ _ _ _ _] -> w312
      event Timeout {
        n152 = event-data() -> ()  [unwired: 1 in, 2 out]
        n153 = Enqueue Element(queue=w319, element=Control_3."main" ("Enum")) -> ()  [unwired: 2 in, 3 out]
      }
      event "Clear subcycle": Value Change {
        n154 = event-data() -> ()  [unwired: 1 in, 5 out]
        n155 = Enqueue Element(queue=w321, element=Control_3."clear table 1" ("Enum")) -> ()  [unwired: 2 in, 3 out]
      }
      event Panel Close? {
        n156 = event-data() -> ()  [unwired: 1 in, 3 out]
        n157 = Two Button Dialog(message="This command will close Eyecat!\nDo you wish to continue?", 1:"No" ("F button name (\"Cancel\")"), 2:"Yes" ("T button name (\"OK\")")) -> (T button?=w323:bool)
        n158 = Not(x=w323) -> (.not. x?=w324:bool)
        n159 = event-data("Discard?"=w324) -> ()  [unwired: 1 in, 1 out]
      }
      event "Save sCycle": Value Change {
        n160 = event-data() -> ()  [unwired: 1 in, 5 out]
        n161 = local read "Sub-Cycle Pattern"() -> (w328:string[][])
        n162 = call "Time column check.vi"("Array"=w328) -> ("Mistake?"=w329:bool)  [unwired: 10 in]
        n163 = case shown="False" w329 {
          tunnel: w330 -> [w332 _]
          frame False {
            n164 = Enqueue Element(queue=w332, element=Control_3."save subc") -> (queue out=w334:refnum<queue>)  [unwired: 2 in, 2 out]
            n165 = Enqueue Element(queue=w334, element=Control_3."update list 1") -> ()  [unwired: 2 in, 3 out]
          }
          frame True {
            n166 = One Button Dialog(message="The time sequence is incorrect!\nReview and save again!") -> ()  [unwired: 1 in, 1 out]
          }
        }
      }
      event "Load sCycle": Value Change {
        n167 = event-data() -> ()  [unwired: 1 in, 5 out]
        n168 = Enqueue Element(queue=w338, element=Control_3."load subc") -> ()  [unwired: 2 in, 3 out]
      }
      event "Delete sCycle": Value Change {
        n169 = event-data() -> ()  [unwired: 1 in, 5 out]
        n170 = Enqueue Element(queue=w345, element=Control_3."delete subc") -> (queue out=w347:refnum<queue>)  [unwired: 2 in, 2 out]
        n171 = Enqueue Element(queue=w347, element=Control_3."update list 1") -> (queue out=w343:refnum<queue>)  [unwired: 2 in, 2 out]
        n172 = Enqueue Element(queue=w343, element=Control_3."update Cycle pattern ") -> (queue out=w340:refnum<queue>)  [unwired: 2 in, 2 out]
        n173 = Enqueue Element(queue=w340, element=Control_3."Total time calc") -> ()  [unwired: 2 in, 3 out]
      }
      event "Sub-Cycle Pattern": Mouse Down; "Sub-Cycle Pattern": Value Change {
        n174 = event-data() -> ()  [unwired: 1 in, 3 out]
        n175 = property on="Sub-Cycle Pattern" class="Tbl (strict)"() -> ("EditPos"=w351:T3)  [unwired: 2 in, 2 out]
        n176 = Unbundle By Name(w351) -> ("Row"=w353:i32)  [unwired: 1 out]
        n177 = Less?(x=w353, y=30) -> (x < y?=w355:bool)
        n178 = case shown="True" w355 {
          tunnel: w352 -> [_ w360]
          frame False {
            n179 = One Button Dialog(message="This table is limited to 30 entries!") -> ()  [unwired: 1 in, 1 out]
          }
          frame True {
            n180 = Enqueue Element(queue=w360, element=Control_3."convert to num") -> (queue out=w359:refnum<queue>)  [unwired: 2 in, 2 out]
            n181 = Enqueue Element(queue=w359, element=Control_3."calc HC CO") -> ()  [unwired: 2 in, 3 out]
          }
        }
        "EditPos Subc" <- w350
        "Flag1" <- TRUE
      }
      event "Clear Cycle Pattern": Value Change {
        n182 = event-data() -> ()  [unwired: 1 in, 5 out]
        n183 = Enqueue Element(queue=w363, element=Control_3."clear table 2" ("Enum")) -> ()  [unwired: 2 in, 3 out]
        n184 = local write "Test Compiled"(FALSE ("Test Compiled")) -> ()
      }
      event "Save Cycle": Value Change {
        n185 = event-data() -> ()  [unwired: 1 in, 5 out]
        n186 = Enqueue Element(queue=w367, element=Control_3."update Cycle pattern ") -> (queue out=w366:refnum<queue>)  [unwired: 2 in, 2 out]
        n187 = Enqueue Element(queue=w366, element=Control_3."save cycle") -> (queue out=w370:refnum<queue>)  [unwired: 2 in, 2 out]
        n188 = Enqueue Element(queue=w370, element=Control_3."update list 2") -> ()  [unwired: 2 in, 3 out]
      }
      event "Load Cycle": Value Change {
        n189 = event-data() -> ()  [unwired: 1 in, 5 out]
        n190 = Enqueue Element(queue=w378, element=Control_3."load cycle") -> (queue out=w376:refnum<queue>)  [unwired: 2 in, 2 out]
        n191 = Enqueue Element(queue=w376, element=Control_3."update Cycle pattern ") -> (queue out=w375:refnum<queue>)  [unwired: 2 in, 2 out]
        n192 = local write "Test Compiled"(FALSE ("Test Compiled")) -> ()
        n193 = Enqueue Element(queue=w375, element=Control_3."Total time calc") -> ()  [unwired: 2 in, 3 out]
      }
      event "Delete Cycle": Value Change {
        n194 = event-data() -> ()  [unwired: 1 in, 5 out]
        n195 = Enqueue Element(queue=w383, element=Control_3."delete cycle") -> (queue out=w382:refnum<queue>)  [unwired: 2 in, 2 out]
        n196 = Enqueue Element(queue=w382, element=Control_3."update list 2") -> ()  [unwired: 2 in, 3 out]
      }
      event Value Change {
        n197 = event-data() -> ()  [unwired: 1 in, 5 out]
        n198 = Enqueue Element(queue=w386, element=Control_3."Total time calc") -> ()  [unwired: 2 in, 3 out]
      }
      event "Cycle Pattern": Mouse Up; "Cycle Pattern": Value Change {
        n199 = event-data() -> ()  [unwired: 1 in, 3 out]
        n200 = property on="Cycle Pattern" class="Tbl (strict)"() -> ("EditPos"=w393:T3)  [unwired: 2 in, 2 out]
        n201 = Unbundle By Name(w393) -> ("Row"=w390:i32, "Column"=w395:i32)
        n202 = Less?(x=w390, y=30) -> (x < y?=w394:bool)
        n203 = case shown="True" w394 {
          tunnel: w395 -> [_ w397]
          tunnel: w391 -> [_ w400]
          frame False {
            n204 = One Button Dialog(message="This table is limited to 30 entries!") -> ()  [unwired: 1 in, 1 out]
          }
          frame True {
            n205 = Equal?(x=w397, y=1) -> (x = y?=w401:bool)
            n206 = case shown="True" w401 {
              tunnel: w400 -> [w404 w407]
              tunnel: [w403 w406] -> w399
              frame False {
                n207 = Enqueue Element(queue=w404, element=Control_3."update Cycle pattern ") -> (queue out=w403:refnum<queue>)  [unwired: 2 in, 2 out]
              }
              frame True {
                n208 = Enqueue Element(queue=w407, element=Control_3."load cycle name") -> (queue out=w406:refnum<queue>)  [unwired: 2 in, 2 out]
              }
            }
            n209 = Enqueue Element(queue=w399, element=Control_3."Total time calc") -> ()  [unwired: 2 in, 3 out]
          }
        }
        "Flag 2" <- TRUE
      }
      event "Compile Test Button": Value Change {
        n210 = event-data() -> ()  [unwired: 1 in, 5 out]
        n211 = local read "Flag 2"() -> (w409:bool)
        n212 = case shown="True" w409 {
          tunnel: w413 -> [w414 w418]
          tunnel: [w414 w415] -> w411
          frame False {
          }
          frame True {
            n213 = Enqueue Element(queue=w418, element=Control_3."save cycle") -> (queue out=w416:refnum<queue>)  [unwired: 2 in, 2 out]
            n214 = Enqueue Element(queue=w416, element=Control_3."update list 2") -> (queue out=w415:refnum<queue>)  [unwired: 2 in, 2 out]
          }
        }
        n215 = Enqueue Element(queue=w411, element=Control_3."load test array") -> ()  [unwired: 2 in, 3 out]
      }
      event Value Change {
        n216 = event-data() -> ()  [unwired: 1 in, 5 out]
        n217 = Enqueue Element(queue=w421, element=Control_3."check scycle name") -> ()  [unwired: 2 in, 3 out]
      }
      event Value Change {
        n218 = event-data() -> ()  [unwired: 1 in, 5 out]
        n219 = Enqueue Element(queue=w422, element=Control_3."check cycle name") -> ()  [unwired: 2 in, 3 out]
      }
      event Value Change {
        n220 = event-data() -> ()  [unwired: 1 in, 5 out]
        n221 = Square(x="Sample Diameter (mm)") -> (x^2=w431:T1)
        n222 = Compound Arithmetic op=MULTIPLY(w431, "Sample Length (mm)", "Number of Samples", 3.141592653589793) -> (w430:T1)
        n223 = Divide(x=w430, y=4000000.0) -> (x/y=→"Sample Volume (litres)":T1)
      }
      event Value Change {
        # "O2Eq"
        n224 = event-data() -> ()  [unwired: 1 in, 5 out]
        n225 = local write "Inlet LAMBDA"("Inlet LAMBDA") -> ()
        n226 = local write "Inlet O2 (%)"("Inlet O2 (%)") -> ()
        n227 = Decrement(x="Inlet LAMBDA") -> (x-1=w446:T1)
        n228 = Multiply(x=4.76, y="Inlet LAMBDA") -> (x*y=w442:T1)
        n229 = Multiply(x=w446, y=100.0) -> (x*y=w444:T1)
        n230 = Add(x=0.33, y=w442) -> (x+y=w440:T1)
        n231 = Divide(x=w444, y=w440) -> (x/y=w439:T1)
        n232 = Subtract(x="Inlet O2 (%)", y=w439) -> (x-y=w437:T1)
        n233 = Multiply(x=w437, y=2.0) -> (x*y=→"CO Theory (%)":T1)
        n234 = Divide(x=w437, y=4.5) -> (x/y=→"HC Theory (%)":T1)
      }
      event Value Change {
        n235 = event-data() -> ()  [unwired: 1 in, 5 out]
        n236 = local write "NO ppm Loff"("NO ppm Loff") -> ()
        n237 = local write "NO:CO Ratio"("NO:CO Ratio") -> ()
        n238 = Divide(x="NO ppm Loff", y=T1 10000.0) -> (x/y=w449:T1)
        n239 = Multiply(x="NO:CO Ratio", y=w449) -> (x*y=→"CO Theory (%)":T1)
      }
      event Value Change {
        n240 = event-data() -> ()  [unwired: 1 in, 5 out]
        n241 = local read "Sample Volume (litres)"() -> (w454:T7)
        n242 = Equal?(x=w454, y=0.0) -> (x = y?=w453:bool)
        n243 = case shown="False" w453 {
          tunnel: w454 -> [w459 _]
          tunnel: "Test Flow Rate(g/s)" -> [w456 _]
          frame False {
            w461 = 60.0 ("y")
            n244 = Multiply(x=w456, y=w461) -> (x*y=w463:T1)
            n245 = Divide(x=w463, y=1.2) -> (x/y=w458:T1)
            "Vol Flow @ STP (l/min)" <- w458
            n246 = Multiply(x=w458, y=w461) -> (x*y=w460:T1)
            n247 = Divide(x=w460, y=w459) -> (x/y=→"Space Velocity (h-1)":T1)
          }
          frame True {
            n248 = One Button Dialog(message="Review sample specification first!") -> ()  [unwired: 1 in, 1 out]
          }
        }
      }
      event "Execute Leak Test Button": Value Change {
        n249 = event-data() -> ()  [unwired: 1 in, 5 out]
        n250 = flat-sequence {
          tunnel: w466 -> [w469]
          tunnel: [w469] -> w465
          tunnel: w465 -> [w472]
          frame #0 {
            n251 = local write "Test number"(u16 5) -> ()
            n252 = local write "Enum 1"(u16 3 ("Test number")) -> ()
          }
          frame #1 {
            n253 = Enqueue Element(queue=w472, element=Control_3."main" ("Enum")) -> (queue out=w470:refnum<queue>)  [unwired: 2 in, 2 out]
            n254 = Enqueue Element(queue=w470, element=Control_3."start test" ("Enum")) -> ()  [unwired: 2 in, 3 out]
          }
        }
      }
      event "Start Test Button": Value Change {
        n255 = event-data() -> ()  [unwired: 1 in, 5 out]
        n256 = property on="Log Test Button" class="Bool (strict)"() -> ("Value"=w477:bool)  [unwired: 2 in, 2 out]
        n257 = Boolean To (0,1)(Boolean=w477) -> (0, 1=w476:i16)
        n258 = Equal To 0?(x=w476) -> (x = 0?=w475:bool)
        n259 = case shown="True" w475 {
          tunnel: [TRUE ("T button?") w480] -> w474
          frame False {
          }
          frame True {
            n260 = Two Button Dialog(message="You are not currently logging data!\nDo you wish to continue?", 1:"No" ("T button name (\"OK\")"), 2:"Yes" ("T button name (\"OK\")")) -> (T button?=w480:bool)
          }
        }
        n261 = case shown="True" w474 {
          tunnel: w478 -> [_ w484]
          frame False {
          }
          frame True {
            n262 = flat-sequence {
              tunnel: w484 -> [w489]
              tunnel: [w489] -> w486
              tunnel: w486 -> [w493]
              tunnel: [w490] -> w485
              tunnel: w485 -> [w501]
              frame #0 {
                n263 = local write "Enum 1"(u16 1 ("Test number")) -> ()
                "Test number" <- "Select Test Type"
              }
              frame #1 {
                n264 = Two Button Dialog(message="Do you wish to connect to\nthe external analyser?   \n") -> (T button?=w491:bool)  [unwired: 2 in]
                n265 = case shown="True" w491 {
                  tunnel: w493 -> [w494 w496]
                  tunnel: [w494 w495] -> w490
                  frame False {
                  }
                  frame True {
                    n266 = Enqueue Element(queue=w496, element=Control_3."Multigas connect" ("Enum")) -> (queue out=w495:refnum<queue>)  [unwired: 2 in, 2 out]
                  }
                }
              }
              frame #2 {
                n267 = Enqueue Element(queue=w501, element=Control_3."main" ("Enum")) -> (queue out=w499:refnum<queue>)  [unwired: 2 in, 2 out]
                n268 = property on="Stop Test Button" class="Bool"("DisabledEnum"=T13."Enabled" ("Disabled")) -> ()  [unwired: 2 in, 2 out]
                n269 = Enqueue Element(queue=w499, element=Control_3."start test" ("Enum")) -> ()  [unwired: 2 in, 3 out]
              }
            }
          }
        }
      }
      event "Log Test Button": Value Change {
        n270 = event-data() -> ()  [unwired: 1 in, 6 out]
        n271 = property on="File Name" class="Str (strict)"() -> ("Value"=w505:T5)  [unwired: 2 in, 2 out]
        n272 = String Length(string=w505) -> (length=w504:i32)
        n273 = Equal To 0?(x=w504) -> (x = 0?=w503:bool)
        n274 = case shown="True" w503 {
          frame False {
          }
          frame True {
            n275 = One Button Dialog(message="A filename has not been entered!") -> ()  [unwired: 1 in, 1 out]
          }
        }
      }
      event "Stop Test Button": Value Change {
        n276 = event-data() -> ()  [unwired: 1 in, 5 out]
        n277 = flat-sequence {
          tunnel: w512 -> [w514]
          tunnel: [w514] -> w511
          tunnel: [w513] -> w509
          tunnel: w511 -> [w518]
          tunnel: [w517] -> w510
          tunnel: w509 -> [w517]
          tunnel: [w516] -> w508
          tunnel: w510 -> [w522]
          tunnel: w508 -> [w521]
          tunnel: [T13."Disabled and Grayed Out" ("Disabled")] -> w507
          frame #0 {
            n278 = local read "Connected?"() -> (w513:bool)
            n279 = local write "Stop Cmd"(T1 1.0 ("Stop Cmd")) -> ()
          }
          frame #1 {
            n280 = Enqueue Element(queue=w518, element=Control_3."main" ("Enum")) -> (queue out=w516:refnum<queue>)  [unwired: 2 in, 2 out]
          }
          frame #2 {
            n281 = case shown="True" w522 {
              tunnel: w521 -> [w523 w526]
              tunnel: [w523 w525] -> _
              frame False {
              }
              frame True {
                n282 = local write "Connected?"(FALSE ("Connected?")) -> ()
                n283 = Enqueue Element(queue=w526, element=Control_3."Multigas disconnect" ("Enum")) -> (queue out=w525:refnum<queue>)  [unwired: 2 in, 2 out]
              }
            }
          }
        }
        n284 = property on="Stop Test Button" class="Bool"("DisabledEnum"=w507) -> ()  [unwired: 2 in, 2 out]
      }
      event "Stopped?": Value Change {
        n285 = event-data() -> ()  [unwired: 1 in, 5 out]
        n286 = flat-sequence {
          tunnel: w530 -> [w534]
          tunnel: [w533] -> w529
          tunnel: [w532] -> w528
          tunnel: w529 -> [w536]
          tunnel: w528 -> [w535]
          frame #0 {
            n287 = local read "Connected?"() -> (w532:bool)
            n288 = Enqueue Element(queue=w534, element=Control_3."main" ("Enum")) -> (queue out=w533:refnum<queue>)  [unwired: 2 in, 2 out]
          }
          frame #1 {
            n289 = case shown="True" w535 {
              tunnel: w536 -> [_ w537]
              frame False {
              }
              frame True {
                n290 = local write "Connected?"(FALSE ("Connected?")) -> ()
                n291 = Enqueue Element(queue=w537, element=Control_3."Multigas disconnect" ("Enum")) -> ()  [unwired: 2 in, 3 out]
              }
            }
          }
        }
      }
      event "Alarm ack": Value Change {
        # "system alarm - set to off"
        n292 = event-data() -> ()  [unwired: 1 in, 5 out]
        n293 = local write "Acknowledge"(TRUE ("Acknowledge")) -> ()
        n294 = property on="Soft Alarm" class="Bool (strict)"("Value"=FALSE ("Acknowledge")) -> ()  [unwired: 2 in, 2 out]
        n295 = property on="Alarm ack" class="Bool"("DisabledEnum"=T13."Disabled and Grayed Out" ("Disabled")) -> ()  [unwired: 2 in, 2 out]
      }
      event "Purge System": Value Change {
        n296 = event-data() -> ()  [unwired: 1 in, 5 out]
        n297 = flat-sequence {
          tunnel: w544 -> [w546]
          tunnel: [w546] -> w543
          tunnel: w543 -> [w547]
          frame #0 {
            n298 = local write "Enum 1"(u16 4 ("Test number")) -> ()
          }
          frame #1 {
            n299 = Enqueue Element(queue=w547, element=Control_3."start test" ("Enum")) -> ()  [unwired: 2 in, 3 out]
          }
        }
      }
      event "Clear log": Value Change {
        n300 = event-data() -> ()  [unwired: 1 in, 5 out]
        n301 = local write "Table"(string[][] [] ("Table")) -> ()
      }
      event "Advanced settings": Value Change {
        # "To be updated"
        # "SO2 conc\nNOx conc\nCO conc\nHC conc\nBleed ratio N2\nBleed ratio CO2"
        n302 = event-data() -> ()  [unwired: 1 in, 5 out]
        n303 = call "Advanced settings MAX.vi"() -> ("output cluster"=→"output cluster":T14)  [unwired: 1 in]
      }
    }
    "stop 2" <- w312
  }
  n304 = while {
    tunnel: w35 -> [w555]
    tunnel: w19 -> [w553]
    tunnel: w21 -> [w552]
    tunnel: [FALSE ("stop 2")] -> w9
    stop <- w556 stop-if-true
    n305 = Dequeue Element(queue=w555) -> (element=w554:T10)  [unwired: 2 in, 3 out]
    n306 = case shown="\"main\", Default" w554 {
      tunnel: w553 -> [_ _ _ w601 w612 w648 w682 _ _ _ _ _ _ _ w1045 _ _ _ _ _ _ _]
      tunnel: w552 -> [_ _ _ _ _ _ _ _ w695 w710 w765 w810 _ _ _ _ _ _ _ _ _ _]
      frame "main", Default {
        # "0 NOx Conc\n1 CO conc %\n2 HC conc %\n3 Bleed H2O \n4 Bleed CO2\n5 Bleed N2 \n6 lambda P\n7 lambda I\n8 lambda D\n9 purge duration\n10 Target furnace lambda\n11 HC reaction ct\n12 Full system\n13 Log interval"
        n307 = local read "output cluster"() -> (w575:T2)
        n308 = Unbundle(w575) -> ("NOx Concentration (ppm)"=w561:T1, "CO concentration %"=w560:T1, "HC concentration %"=w559:T1, "Bleed H2O %"=w558:T1, "Bleed CO2 %"=w557:T1, "Bleed N2 %"=w572:T1, "lambda P"=w571:T1, "lambda I"=w570:T1, "lambda D"=w573:T1, "Purge duration (seconds)"=w574:T1, "Target furnace lambda"=w566:T1, "HC reaction constant"=w565:T1, w567:i16, "Log interval (HRS)"=→"Log interval (seconds)":T1)
        n309 = local read "Test Flow Rate(g/s)"() -> (w587:T1)
        n310 = local read "Test number"() -> (w592:u16)
        n311 = local read "Connected?"() -> (w581:bool)
        n312 = local read "NO ppm Loff"() -> (w577:T1)
        n313 = local read "NO:CO Ratio"() -> (w576:T1)
        n314 = local read "Inlet LAMBDA"() -> (w579:T1)
        n315 = local read "Inlet O2 (%)"() -> (w578:T1)
        n316 = Boolean To (0,1)(Boolean=w581) -> (0, 1=w564:i16)
        n317 = Not Equal To 0?(x=w567) -> (x != 0?=→"Full system?":bool)
        n318 = Build Array("Stop Cmd", w592, w587, "Test Start Temperature (°C)", "Test Stop temperature (°C)", "Furnace Ramp Rate (°C/min)", w579, w578, "Inlet LAMBDA Rich", "Inlet LAMBDA Lean", "Inlet Temperature (°C)", "NO ppm SW", w577, w576, "Temperature Limit (°C)", w564, "Inlet temp Age", "Flow rate Age", w561, w560, w559, w558, w557, w572, w571, w570, w573, w574, w566, w565, w567) -> (w583:T1[])
        n319 = shared-variable "NI-cRIO9074-018C1D8D\\Library 1.lvlib\\Control Variables"(w583) -> ()  [unwired: 1 in, 1 out]
      }
      frame "start test" {
        w593 = FALSE
        n320 = property on="Pass" class="Bool (strict)"("Value"=w593) -> ()  [unwired: 2 in, 2 out]
        n321 = property on="Fail" class="Bool (strict)"("Value"=w593) -> ()  [unwired: 2 in, 2 out]
        n322 = local write "Pass"(w593) -> ()
        n323 = local write "Fail"(w593) -> ()
        n324 = shared-variable "NI-cRIO9074-018C1D8D\\Library 1.lvlib\\Enum 1"("Enum 1") -> ()  [unwired: 1 in, 1 out]
      }
      frame "clear table 1" {
        n325 = property on="Sub-Cycle Name" class="Str (strict)"("Value"="" ("Subcycle name")) -> ()  [unwired: 2 in, 2 out]
        n326 = local write "Flag1"(FALSE) -> ()
        n327 = local write "Sub-Cycle Pattern"(string[][] [["", "0", "", "", "", "", "", "", "", "", "", "", ""], ["", "", "", "", "", "", "", "", "", "", "", "", ""], ["", "", "", "", "", "", "", "", "", "", "", "", ""], ["", "", "", "", "", "", "", "", "", "", "", "", ""], ["", "", "", "", "", "", "", "", "", "", "", "", ""], ["", "", "", "", "", "", "", "", "", "", "", "", ""], ["", "", "", "", "", "", "", "", "", "", "", "", ""], ["", "", "", "", "", "", "", "", "", "", "", "", ""], ["", "", "", "", "", "", "", "", "", "", "", "", ""], ["", "", "", "", "", "", "", "", "", "", "", "", ""], ["", "", "", "", "", "", "", "", "", "", "", "", ""], ["", "", "", "", "", "", "", "", "", "", "", "", ""], ["", "", "", "", "", "", "", "", "", "", "", "", ""], ["", "", "", "", "", "", "", "", "", "", "", "", ""], ["", "", "", "", "", "", "", "", "", "", "", "", ""], ["", "", "", "", "", "", "", "", "", "", "", "", ""], ["", "", "", "", "", "", "", "", "", "", "", "", ""], ["", "", "", "", "", "", "", "", "", "", "", "", ""], ["", "", "", "", "", "", "", "", "", "", "", "", ""], ["", "", "", "", "", "", "", "", "", "", "", "", ""], ["", "", "", "", "", "", "", "", "", "", "", "", ""], ["", "", "", "", "", "", "", "", "", "", "", "", ""], ["", "", "", "", "", "", "", "", "", "", "", "", ""], ["", "", "", "", "", "", "", "", "", "", "", "", ""], ["", "", "", "", "", "", "", "", "", "", "", "", ""], ["", "", "", "", "", "", "", "", "", "", "", "", ""], ["", "", "", "", "", "", "", "", "", "", "", "", ""], ["", "", "", "", "", "", "", "", "", "", "", "", ""], ["", "", "", "", "", "", "", "", "", "", "", "", ""], ["", "", "", "", "", "", "", "", "", "", "", "", ""], ["", "", "", "", "", "", "", "", "", "", "", "", ""]]) -> ()
      }
      frame "update list 1" {
        n328 = String To Path(string=w601) -> (path=w600:path)
        n329 = List Folder(path=w600, pattern="*.eyes") -> (filenames=w599:string[])  [unwired: 2 in, 3 out]
        n330 = property on="Sub-Cycle List" class="LstBox (strict)"("Item Names"=w599) -> ()  [unwired: 2 in, 2 out]
      }
      frame "save subc" {
        w605 = ".eyes" ("string")
        n331 = local read "Sub-Cycle Name"() -> (w604:T5)
        n332 = String To Path(string=w612) -> (path=w617:path)
        n333 = Equal?(x=w604, y="") -> (x = y?=w609:bool)
        n334 = List Folder(path=w617, pattern="*.eyes" ("string")) -> (filenames=w616:string[])  [unwired: 2 in, 3 out]
        n335 = Concatenate Strings(w604, w605) -> (w603:string)
        n336 = Concatenate Strings(w612, w604, w605) -> (w618:string)
        n337 = Search 1D Array(1D array=w616, element=w603) -> (index of element=w615:i32)  [unwired: 1 in]
        n338 = case shown="True" w609 {
          tunnel: [TRUE FALSE] -> w608
          frame False {
          }
          frame True {
            n339 = One Button Dialog(message="Insert file name!") -> ()  [unwired: 1 in, 1 out]
          }
        }
        n340 = String To Path(string=w618) -> (path=w611:path)
        n341 = Equal?(x=w615, y=-1) -> (x = y?=w613:bool)
        n342 = case shown="False" w613 {
          selector: w613 -> [_ w624]
          tunnel: [w622 w624] -> w607
          frame False {
            n343 = Two Button Dialog(message="A file with this name already exists!\nDo you want to overwrite?") -> (T button?=w622:bool)  [unwired: 2 in]
          }
          frame True {
          }
        }
        n344 = And(x=w607, y=w608) -> (x .and. y?=w606:bool)
        n345 = case shown="True" w606 {
          tunnel: w611 -> [_ w629]
          frame False {
          }
          frame True {
            n346 = local read "Sub-Cycle Pattern"() -> (w628:string[][])
            n347 = call "Table check.vi"("Input table"=w628) -> ("Incomplete?"=w626:bool, "Length"=w627:i32)  [unwired: 9 in]
            n348 = case shown="False" w626 {
              tunnel: w628 -> [w637 _]
              tunnel: w629 -> [w636 _]
              tunnel: w627 -> [w635 _]
              tunnel: string[] [] -> [w634 _]
              frame False {
                n349 = for {
                  N: w635 -> [_]
                  tunnel: w637 -> [w644]
                  shift-right: [w641] -> w633
                  shift-left: w634 -> [w642]
                  i -> [w643]
                  n350 = Index Array(array=w644, index (row)=w643) -> (element=w640:string[])  [unwired: 1 in]
                  n351 = Delete From Array(array=w640, index=0) -> (array with subset deleted=w639:string[])  [unwired: 1 in, 1 out]
                  n352 = Build Array (concatenate)(w642, w639) -> (w641:string[])
                }
                n353 = Build Array (concatenate)("SubCycle Data File for EYECAT - do not modify", w633) -> (w631:string[])
                n354 = call-poly <vilib>:"Write To Spreadsheet File.vi"("1D data"=w631, "file path (dialog if empty)"=w636) -> ()  [unwired: 6 in, 1 out]
              }
              frame True {
                n355 = One Button Dialog(message="The table is incomplete!\nplease review and save again!") -> ()  [unwired: 1 in, 1 out]
              }
            }
            n356 = local write "Flag1"(FALSE) -> ()
          }
        }
      }
      frame "load subc" {
        n357 = local read "Flag1"() -> (w649:bool)
        n358 = case shown="True" w649 {
          tunnel: [w676 w678] -> w647
          tunnel: w648 -> [w676 w678]
          tunnel: [TRUE w677] -> w646
          frame False {
          }
          frame True {
            n359 = Two Button Dialog(message="The table has been modified.\nDo you want to continue?") -> (T button?=w677:bool)  [unwired: 2 in]
          }
        }
        n360 = case shown="True" w646 {
          tunnel: w647 -> [_ w653]
          frame False {
          }
          frame True {
            n361 = property on="Sub-Cycle List" class="LstBox (strict)"() -> ("Item Names"=w665:string[])  [unwired: 2 in, 2 out]
            n362 = Index Array(array=w665, index="Sub-Cycle List") -> (element=w652:string)
            n363 = Concatenate Strings(w653, w652) -> (w663:string)
            n364 = Search/Split String(string=w652, search string/char (-)=".") -> (substring before match=w650:string)  [unwired: 1 in, 2 out]
            n365 = local write "Sub-Cycle Name"(w650) -> ()
            n366 = String To Path(string=w663) -> (path=w662:path)
            n367 = call-poly <vilib>:"Read From Spreadsheet File.vi"("file path (dialog if empty)"=w662) -> ("first row"=w658:string[])  [unwired: 6 in, 4 out]
            n368 = Delete From Array(array=w658, length=1, index=0) -> (array with subset deleted=w655:string[])  [unwired: 1 out]
            n369 = Array Size(array=w655) -> (size(s)=w661:i32)
            n370 = Divide(x=w661, y=12) -> (x/y=w654:dbl)
            n371 = for {
              N: w654 -> [_]
              shift-right: [w671] -> _
              shift-left: w655 -> [w674]
              tunnel: [w670] -> w659 mode=indexing
              i -> [w669]
              n372 = Increment(x=w669) -> (x+1=w668:i32)
              n373 = Delete From Array(array=w674, length=12, index=0) -> (deleted portion=w666:string[], array with subset deleted=w671:string[])
              n374 = Number To Decimal String(number=w668) -> (decimal integer string=w667:string)  [unwired: 1 in]
              n375 = Build Array (concatenate)(w667, w666) -> (w670:string[])
            }
            n376 = local write "Sub-Cycle Pattern"(w659) -> ()
          }
        }
      }
      frame "delete subc" {
        n377 = Two Button Dialog(message="This operation will permanently delete this file!\nDo you want to continue?") -> (T button?=w681:bool)  [unwired: 2 in]
        n378 = case shown="True" w681 {
          tunnel: w682 -> [_ w687]
          frame False {
          }
          frame True {
            n379 = local read "Sub-Cycle List"() -> (w684:i32)
            n380 = property on="Sub-Cycle List" class="LstBox (strict)"() -> ("Item Names"=w685:string[])  [unwired: 2 in, 2 out]
            n381 = Index Array(array=w685, index=w684) -> (element=w689:string)
            n382 = Concatenate Strings(w687, w689) -> (w688:string)
            n383 = local write "Flag1"(FALSE) -> ()
            n384 = String To Path(string=w688) -> (path=w686:path)
            n385 = Delete(path (use dialog)=w686) -> ()  [unwired: 4 in, 3 out]
          }
        }
      }
      frame "clear table 2" {
        n386 = property on="Cycle Name" class="Str (strict)"("Value"="" ("Subcycle name")) -> ()  [unwired: 2 in, 2 out]
        n387 = local write "Flag 2"(FALSE) -> ()
        n388 = local write "Cycle Pattern"(string[][] [["", "", "", "", ""], ["", "", "", "", ""], ["", "", "", "", ""], ["", "", "", "", ""], ["", "", "", "", ""], ["", "", "", "", ""], ["", "", "", "", ""], ["", "", "", "", ""], ["", "", "", "", ""], ["", "", "", "", ""], ["", "", "", "", ""], ["", "", "", "", ""], ["", "", "", "", ""], ["", "", "", "", ""], ["", "", "", "", ""], ["", "", "", "", ""], ["", "", "", "", ""], ["", "", "", "", ""], ["", "", "", "", ""], ["", "", "", "", ""], ["", "", "", "", ""], ["", "", "", "", ""], ["", "", "", "", ""], ["", "", "", "", ""], ["", "", "", "", ""], ["", "", "", "", ""], ["", "", "", "", ""], ["", "", "", "", ""], ["", "", "", "", ""], ["", "", "", "", ""], ["", "", "", "", ""]]) -> ()
      }
      frame "update list 2" {
        n389 = String To Path(string=w695) -> (path=w696:path)
        n390 = List Folder(path=w696, pattern="*.eyec") -> (filenames=w694:string[])  [unwired: 2 in, 3 out]
        n391 = property on="Cycle List" class="LstBox (strict)"("Item Names"=w694) -> ()  [unwired: 2 in, 2 out]
      }
      frame "save cycle" {
        w697 = ".eyec" ("string")
        n392 = local read "Cycle Name"() -> (w698:T5)
        n393 = String To Path(string=w710) -> (path=w711:path)
        n394 = List Folder(path=w711, pattern="*.eyec" ("string")) -> (filenames=w709:string[])  [unwired: 2 in, 3 out]
        n395 = Equal?(x=w698, y="") -> (x = y?=w704:bool)
        n396 = Concatenate Strings(w698, w697) -> (w700:string)
        n397 = Search 1D Array(1D array=w709, element=w700) -> (index of element=w708:i32)  [unwired: 1 in]
        n398 = Concatenate Strings(w710, w698, w697) -> (w713:string)
        n399 = case shown="True" w704 {
          tunnel: [TRUE FALSE] -> w702
          frame False {
          }
          frame True {
            n400 = One Button Dialog(message="Insert file name!") -> ()  [unwired: 1 in, 1 out]
          }
        }
        n401 = String To Path(string=w713) -> (path=w712:path)
        n402 = Equal?(x=w708, y=-1) -> (x = y?=w706:bool)
        n403 = case shown="False" w706 {
          selector: w706 -> [_ w762]
          tunnel: [w760 w762] -> w703
          frame False {
            n404 = Two Button Dialog(message="A file with this name already exists!\nDo you want to overwrite?") -> (T button?=w760:bool)  [unwired: 2 in]
          }
          frame True {
          }
        }
        n405 = And(x=w703, y=w702) -> (x .and. y?=w701:bool)
        n406 = case shown="True" w701 {
          tunnel: w712 -> [_ w720]
          frame False {
          }
          frame True {
            n407 = local read "Cycle Pattern"() -> (w719:string[][])
            n408 = call "Table check.vi"("Input table"=w719) -> ("Incomplete?"=w717:bool, "Length"=w718:i32)  [unwired: 9 in]
            n409 = case shown="False" w717 {
              tunnel: w720 -> [w729 _]
              tunnel: w719 -> [w728 _]
              tunnel: w718 -> [w721 _]
              frame False {
                n410 = Number To Decimal String(number=w721) -> (decimal integer string=w724:string)  [unwired: 1 in]
                n411 = for {
                  N: w721 -> [_]
                  tunnel: w728 -> [w758]
                  shift-right: [w746] -> w725
                  shift-left: string[] [] -> [w756]
                  i -> [w757]
                  w737 = 12 ("length")
                  n412 = Index Array(array=w758, index (row)=w757) -> (element=w752:string[])  [unwired: 1 in]
                  n413 = Index Array(array=w752, index=3) -> (element=w742:string)
                  n414 = Index Array(array=w752, index=1) -> (element=w741:string)
                  n415 = Concatenate Strings("C:\\Setup Files\\Subcycles Folder\\", w741) -> (w753:string)
                  n416 = String To Path(string=w753) -> (path=w754:path)
                  n417 = call-poly <vilib>:"Read From Spreadsheet File.vi"("file path (dialog if empty)"=w754) -> ("first row"=w745:string[])  [unwired: 6 in, 4 out]
                  n418 = Delete From Array(array=w745, length=1, index=0) -> (array with subset deleted=w739:string[])  [unwired: 1 out]
                  n419 = String Length(string=w739) -> (length=w748:i32[])
                  n420 = Array Size(array=w748) -> (size(s)=w740:i32)
                  n421 = Divide(x=w740, y=w737) -> (x/y=w738:dbl)
                  n422 = Decrement(x=w738) -> (x-1=w730:dbl)
                  n423 = Multiply(x=w737, y=w730) -> (x*y=w736:dbl)
                  n424 = Number To Decimal String(number=w730) -> (decimal integer string=w747:string)  [unwired: 1 in]
                  n425 = Delete From Array(array=w739, length=12, index=w736) -> (deleted portion=w733:string[], array with subset deleted=w734:string[])
                  n426 = Index Array(array=w733, index=0) -> (element=w731:string)
                  n427 = Build Array (concatenate)(w741, w742, w747, w731, w734) -> (w751:string[])
                  n428 = Build Array (concatenate)(w756, w751) -> (w746:string[])
                }
                n429 = local write "Flag 2"(FALSE) -> ()
                n430 = Build Array (concatenate)("Cycle Data File for EYECAT - do not modify", w724, w725) -> (w726:string[])
                n431 = call-poly <vilib>:"Write To Spreadsheet File.vi"("1D data"=w726, "file path (dialog if empty)"=w729) -> ()  [unwired: 6 in, 1 out]
              }
              frame True {
                n432 = One Button Dialog(message="The table is incomplete!\nplease review and save again!") -> ()  [unwired: 1 in, 1 out]
              }
            }
          }
        }
      }
      frame "load cycle" {
        n433 = local read "Flag 2"() -> (w766:bool)
        n434 = case shown="True" w766 {
          tunnel: [w805 w807] -> w763
          tunnel: w765 -> [w805 w807]
          tunnel: [TRUE ("T button?") w806] -> w764
          frame False {
          }
          frame True {
            n435 = Two Button Dialog(message="The table has been modified.\nDo you want to continue?") -> (T button?=w806:bool)  [unwired: 2 in]
          }
        }
        n436 = case shown="True" w764 {
          tunnel: w763 -> [_ w769]
          frame False {
          }
          frame True {
            n437 = property on="Cycle List" class="LstBox (strict)"() -> ("Item Names"=w785:string[])  [unwired: 2 in, 2 out]
            n438 = Index Array(array=w785, index="Cycle List") -> (element=w771:string)
            n439 = Concatenate Strings(w769, w771) -> (w784:string)
            n440 = Search/Split String(string=w771, search string/char (-)=".") -> (substring before match=w770:string)  [unwired: 1 in, 2 out]
            n441 = String To Path(string=w784) -> (path=w783:path)
            n442 = local write "Cycle Name"(w770) -> ()
            n443 = call-poly <vilib>:"Read From Spreadsheet File.vi"("file path (dialog if empty)"=w783) -> ("first row"=w767:string[])  [unwired: 6 in, 4 out]
            n444 = Delete From Array(array=w767, length=2, index=0) -> (array with subset deleted=w768:string[])  [unwired: 1 out]
            n445 = Index Array(array=w767, index=1) -> (element=w782:string)
            n446 = Decimal String To Number(string=w782) -> (number=w781:i32)  [unwired: 2 in, 1 out]
            n447 = for {
              N: w781 -> [_]
              tunnel: w768 -> [w803]
              tunnel: [w798] -> w776 mode=indexing
              shift-right: [w788] -> _
              shift-left: 0 ("x") -> [w789]
              i -> [w802]
              w799 = ""
              n448 = Increment(x=w789) -> (x+1=w787:i32)
              n449 = Increment(x=w787) -> (x+1=w795:i32)
              n450 = Increment(x=w802) -> (x+1=w797:i32)
              n451 = Number To Decimal String(number=w797) -> (decimal integer string=w796:string)  [unwired: 1 in]
              n452 = Index Array(array=w803, index #1=w789, index #2=w787, index #3=w795) -> (element #1=w801:string, element #2=w800:string, element #3=w794:string)
              n453 = Build Array(w796, w801, w799, w800, w799) -> (w798:string[])
              n454 = Decimal String To Number(string=w794) -> (number=w793:i32)  [unwired: 2 in, 1 out]
              n455 = Multiply(x=w793, y=12 ("x")) -> (x*y=w791:i32)
              n456 = Compound Arithmetic op=ADD(w791, 4, w789) -> (w788:i32)
            }
            n457 = Insert Into Array(array=string[][] [["", "", "", "", ""], ["", "", "", "", ""], ["", "", "", "", ""], ["", "", "", "", ""], ["", "", "", "", ""], ["", "", "", "", ""], ["", "", "", "", ""], ["", "", "", "", ""], ["", "", "", "", ""], ["", "", "", "", ""], ["", "", "", "", ""], ["", "", "", "", ""], ["", "", "", "", ""], ["", "", "", "", ""], ["", "", "", "", ""], ["", "", "", "", ""], ["", "", "", "", ""], ["", "", "", "", ""], ["", "", "", "", ""], ["", "", "", "", ""], ["", "", "", "", ""], ["", "", "", "", ""], ["", "", "", "", ""], ["", "", "", "", ""], ["", "", "", "", ""], ["", "", "", "", ""], ["", "", "", "", ""], ["", "", "", "", ""], ["", "", "", "", ""], ["", "", "", "", ""], ["", "", "", "", ""]], index (row)=0, new element=w776) -> (w775:string[][])  [unwired: 1 in]
            n458 = local write "Cycle Pattern"(w775) -> ()
          }
        }
      }
      frame "delete cycle" {
        n459 = Two Button Dialog(message="This operation will permanently delete this file!\nDo you want to continue?") -> (T button?=w811:bool)  [unwired: 2 in]
        n460 = case shown="True" w811 {
          tunnel: w810 -> [_ w816]
          frame False {
          }
          frame True {
            n461 = local read "Cycle List"() -> (w817:i32)
            n462 = property on="Cycle List" class="LstBox (strict)"() -> ("Item Names"=w818:string[])  [unwired: 2 in, 2 out]
            n463 = Index Array(array=w818, index=w817) -> (element=w815:string)
            n464 = Concatenate Strings(w816, w815) -> (w814:string)
            n465 = String To Path(string=w814) -> (path=w813:path)
            n466 = Delete(path (use dialog)=w813) -> ()  [unwired: 4 in, 3 out]
            n467 = local write "Flag 2"(FALSE) -> ()
          }
        }
      }
      frame "calc HC CO" {
        n468 = local read "Sub-Cycle Pattern"() -> (w835:string[][])
        n469 = Index Array(array=w835, index (col) #1=3 ("disabled index (col)"), index (col) #2=4 ("index (col)"), index (col) #3=11 ("index (col)")) -> (element #1=w825:string[], element #2=w832:string[], element #3=w819:string[])  [unwired: 3 in]
        n470 = Array Size(array=w825) -> (size(s)=w823:i32)
        n471 = Search 1D Array(1D array=w825, element="") -> (index of element=w822:i32)  [unwired: 1 in]
        n472 = Equal?(x=w822, y=-1) -> (x = y?=w824:bool)
        n473 = Select(t=w823, s=w824, f=w822) -> (s? t:f=w821:i32)
        n474 = for {
          N: w821 -> [_]
          tunnel: [w846] -> w829 mode=indexing
          tunnel: [w845] -> w828 mode=indexing
          tunnel: w825 -> [w844] mode=indexing
          tunnel: w832 -> [w843] mode=indexing
          tunnel: w819 -> [w842] mode=indexing
          w841 = ""
          n475 = Not Equal?(x=w844, y=w841) -> (x != y?=w840:bool)
          n476 = Not Equal?(x=w843, y=w841) -> (x != y?=w839:bool)
          n477 = Not Equal?(x=w842, y=w841) -> (x != y?=w838:bool)
          n478 = Compound Arithmetic op=AND(w840, w839, w838) -> (w837:bool)
          n479 = case shown="True" w837 {
            tunnel: w844 -> [_ w875]
            tunnel: w843 -> [_ w874]
            tunnel: [w847 w871] -> w845
            tunnel: [w847 w870] -> w846
            tunnel: w842 -> [_ w848]
            frame False {
              w847 = ""
            }
            frame True {
              # "O2Eq"
              n480 = Fract/Exp String To Number(string=w848) -> (number=w849:dbl)  [unwired: 3 in, 1 out]
              n481 = Fract/Exp String To Number(string=w875) -> (number=w856:dbl)  [unwired: 3 in, 1 out]
              n482 = Fract/Exp String To Number(string=w874) -> (number=w852:dbl)  [unwired: 3 in, 1 out]
              n483 = Decrement(x=w856) -> (x-1=w857:dbl)
              n484 = Divide(x=w849, y=20000.0) -> (x/y=w850:dbl)
              n485 = Multiply(x=4.76, y=w856) -> (x*y=w861:dbl)
              n486 = Multiply(x=w857, y=100.0) -> (x*y=w859:dbl)
              n487 = Add(x=w852, y=w850) -> (x+y=w853:dbl)
              n488 = Add(x=0.33, y=w861) -> (x+y=w863:dbl)
              n489 = Divide(x=w859, y=w863) -> (x/y=w864:dbl)
              n490 = Subtract(x=w853, y=w864) -> (x-y=w866:dbl)
              n491 = Multiply(x=w866, y=2.0) -> (x*y=w854:dbl)
              n492 = Divide(x=w866, y=5.0) -> (x/y=w855:dbl)
              n493 = Number To Fractional String(number=w855, width (-)=i16 6, precision (6)=i16 3) -> (F-format string=w870:string)  [unwired: 1 in]
              n494 = Number To Fractional String(number=w854, width (-)=i16 6, precision (6)=i16 2) -> (F-format string=w871:string)  [unwired: 1 in]
            }
          }
        }
        n495 = Replace Array Subset(array=w835, new element #1=w829, index (col) #1=5 ("disabled index (col)"), new element #2=w828, index (col) #2=6 ("disabled index (col)")) -> (w833:string[][])  [unwired: 2 in]
        n496 = local write "Sub-Cycle Pattern"(w833) -> ()
      }
      frame "Total time calc" {
        w890 = i16 2 ("width (-)")
        w897 = ":"
        n497 = local read "Cycle Pattern"() -> (w904:string[][])
        n498 = Index Array(array=w904, index (col)=4 ("disabled index (col)")) -> (element=w877:string[])  [unwired: 1 in]
        n499 = Array Size(array=w877) -> (size(s)=w879:i32)
        n500 = Search 1D Array(1D array=w877, element="") -> (index of element=w878:i32)  [unwired: 1 in]
        n501 = Equal?(x=w878, y=-1) -> (x = y?=w880:bool)
        n502 = Select(t=w879, s=w880, f=w878) -> (s? t:f=w876:i32)
        n503 = for {
          N: w876 -> [_]
          tunnel: w877 -> [w912] mode=indexing
          shift-right: [w914] -> w900
          shift-left: 0 -> [w915]
          n504 = xnode "Match Regular Expression"("input string"=w912, "regular expression"=":" ("search string/char (-)")) -> ("before match"=w911:string, "after match"=w908:string)  [unwired: 4 in, 3 out]
          n505 = Decimal String To Number(string=w911) -> (number=w910:i32)  [unwired: 2 in, 1 out]
          n506 = Decimal String To Number(string=w908) -> (number=w907:i32)  [unwired: 2 in, 1 out]
          n507 = Multiply(x=w910, y=60) -> (x*y=w906:i32)
          n508 = Add(x=w906, y=w907) -> (x+y=w905:i32)
          n509 = Add(x=w905, y=w915) -> (x+y=w914:i32)
        }
        n510 = local read "Total Number of Cycles"() -> (w901:T1)
        n511 = Multiply(x=w900, y=w901) -> (x*y=w896:T1)
        n512 = Quotient & Remainder(x=w896, y=3600.0) -> (x-y*floor(x/y)=w883:T1, floor(x/y)=w893:T1)
        n513 = Quotient & Remainder(x=w883, y=60.0) -> (x-y*floor(x/y)=w891:T1, floor(x/y)=w892:T1)
        n514 = Number To Decimal String(number=w893) -> (decimal integer string=w898:string)  [unwired: 1 in]
        n515 = Number To Decimal String(number=w892, width (-)=w890) -> (decimal integer string=w894:string)
        n516 = Number To Decimal String(number=w891, width (-)=w890) -> (decimal integer string=w889:string)
        n517 = Concatenate Strings(w898, w897, w894, w897, w889) -> (w888:string)
        n518 = call <vilib>:"Search and Replace Pattern.vi"("string"=w888, "regular expression (\"\")"=" " ("replace string (\"\")"), "replace string (\"\")"="0" ("replace string (\"\")"), "replace all? (F)"=TRUE) -> ("result string"=→"Total Test Duration (hrs)":string)  [unwired: 1 in, 1 out]
      }
      frame "update Cycle pattern " {
        n519 = local read "Cycle Pattern"() -> (w1043:string[][])
        n520 = Index Array(array=w1043, index (col)=1 ("disabled index (col)")) -> (element=w1028:string[])  [unwired: 1 in]
        n521 = String To Path(string=w1045) -> (path=w1046:path)
        n522 = Array Size(array=w1028) -> (size(s)=w1031:i32)
        n523 = Search 1D Array(1D array=w1028, element="") -> (index of element=w1030:i32)  [unwired: 1 in]
        n524 = List Folder(path=w1046, pattern="*.eyes") -> (filenames=w1044:string[])  [unwired: 2 in, 3 out]
        n525 = Equal?(x=w1030, y=-1) -> (x = y?=w1032:bool)
        n526 = Select(t=w1031, s=w1032, f=w1030) -> (s? t:f=w1029:i32)
        n527 = for {
          N: w1029 -> [_]
          tunnel: w1043 -> [w1062] mode=indexing
          tunnel: w1045 -> [w1055]
          tunnel: [w1057] -> w1038 mode=indexing
          tunnel: [w1059] -> w1042 mode=indexing
          tunnel: [w1056] -> w1039 mode=indexing
          tunnel: w1044 -> [w1054]
          tunnel: [w1049] -> w1035 mode=indexing
          n528 = Index Array(array=w1062, index #1=1 ("index"), index #2=3 ("index")) -> (element #1=w1053:string, element #2=w1058:string)
          n529 = Search 1D Array(1D array=w1054, element=w1053) -> (index of element=w1052:i32)  [unwired: 1 in]
          n530 = Not Equal?(x=w1052, y=-1) -> (x != y?=w1050:bool)
          n531 = case shown="True" w1050 {
            tunnel: [w1066 w1080] -> w1059
            tunnel: w1058 -> [_ w1076]
            tunnel: [w1066 w1074] -> w1057
            tunnel: [w1066 w1073] -> w1056
            tunnel: w1055 -> [_ w1072]
            tunnel: w1053 -> [w1065 w1071]
            tunnel: [w1064 w1071] -> w1049
            frame False {
              w1066 = "N/A" ("String")
              n532 = Concatenate Strings(w1065, " - File NOT AVAILABLE !!!" ("string")) -> (w1064:string)
            }
            frame True {
              w1084 = i16 2 ("width (-)")
              n533 = Concatenate Strings(w1072, w1071) -> (w1102:string)
              n534 = String To Path(string=w1102) -> (path=w1101:path)
              n535 = call <vilib>:"Search and Replace Pattern.vi"("string"=w1076, "regular expression (\"\")"="[a-x ]" ("format string"), "replace string (\"\")"="", "replace all? (F)"=TRUE) -> ("result string"=w1073:string)  [unwired: 1 in, 1 out]
              n536 = call-poly <vilib>:"Read From Spreadsheet File.vi"("file path (dialog if empty)"=w1101) -> ("first row"=w1070:string[])  [unwired: 6 in, 4 out]
              n537 = Delete From Array(array=w1070, length=1, index=0) -> (array with subset deleted=w1069:string[])  [unwired: 1 out]
              n538 = Array Size(array=w1069) -> (size(s)=w1100:i32)
              n539 = Equal?(x=w1073, y="") -> (x = y?=w1088:bool)
              n540 = Subtract(x=w1100, y=12) -> (x-y=w1098:i32)
              n541 = Select(t="0", s=w1088, f=w1073) -> (s? t:f=w1087:string)
              n542 = Index Array(array=w1069, index=w1098) -> (element=w1074:string)
              n543 = Decimal String To Number(string=w1087) -> (number=w1097:i32)  [unwired: 2 in, 1 out]
              n544 = Decimal String To Number(string=w1074) -> (number=w1096:i32)  [unwired: 2 in, 1 out]
              n545 = Multiply(x=w1097, y=w1096) -> (x*y=w1095:i32)
              n546 = Quotient & Remainder(x=w1095, y=60) -> (x-y*floor(x/y)=w1093:i32, floor(x/y)=w1092:i32)
              n547 = Number To Decimal String(number=w1093, width (-)=w1084) -> (decimal integer string=w1090:string)
              n548 = Number To Decimal String(number=w1092, width (-)=w1084) -> (decimal integer string=w1089:string)
              n549 = Concatenate Strings(w1089, ":", w1090) -> (w1083:string)
              n550 = call <vilib>:"Search and Replace Pattern.vi"("string"=w1083, "regular expression (\"\")"=" " ("replace string (\"\")"), "replace string (\"\")"="0" ("replace string (\"\")"), "replace all? (F)"=TRUE) -> ("result string"=w1080:string)  [unwired: 1 in, 1 out]
            }
          }
        }
        n551 = Replace Array Subset(array=w1043, new element #1=w1035, index (col) #1=1 ("disabled index (col)"), new element #2=w1038, index (col) #2=2 ("disabled index (col)"), new element #3=w1039, index (col) #3=3 ("disabled index (col)"), new element #4=w1042, index (col) #4=4 ("disabled index (col)")) -> (w1047:string[][])  [unwired: 4 in]
        n552 = local write "Cycle Pattern"(w1047) -> ()
      }
      frame "load cycle name" {
        n553 = property on="Cycle Pattern" class="Tbl (strict)"() -> ("EditPos"=w1108:T3)  [unwired: 2 in, 2 out]
        n554 = Unbundle By Name(w1108) -> ("Row"=w1106:i32, "Column"=w1105:i32)
        n555 = local read "Cycle Pattern"() -> (w1104:string[][])
        n556 = call "SubCycles list.vi"() -> ("Subcycle name"=w1107:string)  [unwired: 10 in, 1 out]
        n557 = Replace Array Subset(array=w1104, new element=w1107, index (row)=w1106, index (col)=w1105) -> (w1103:string[][])
        n558 = local write "Cycle Pattern"(w1103) -> ()
      }
      frame "load test array" {
        n559 = local read "Total Test Duration (hrs)"() -> (w1116:T8)
        n560 = local read "Cycle Name"() -> (w1112:T5)
        n561 = Equal?(x=w1112, y="") -> (x = y?=w1111:bool)
        n562 = Not Equal?(x=w1116, y="0:00:00") -> (x != y?=w1110:bool)
        n563 = Or(x=w1110, y=w1111) -> (x .or. y?=w1109:bool)
        n564 = case shown="True" w1109 {
          selector: w1109 -> [w1117 _]
          tunnel: [FALSE TRUE] -> w1114
          frame False {
            n565 = case shown="False" w1117 {
              frame False {
                n566 = One Button Dialog(message="Incomplete Data!\nReview the cycle pattern!") -> ()  [unwired: 1 in, 1 out]
              }
              frame True {
              }
            }
          }
          frame True {
            w1123 = 0.0 ("default (0 I32)")
            n567 = local read "Cycle Name"() -> (w1138:T5)
            n568 = Concatenate Strings("C:\\Setup Files\\Cycles Folder\\", w1138, ".eyec" ("string")) -> (w1136:string)
            n569 = String To Path(string=w1136) -> (path=w1137:path)
            n570 = local read "Total Number of Cycles"() -> (w1134:T1)
            n571 = call-poly <vilib>:"Read From Spreadsheet File.vi"("file path (dialog if empty)"=w1137) -> ("first row"=w1120:string[])  [unwired: 6 in, 4 out]
            n572 = call "Remove names.vi"("Array in"=w1120) -> ("Array out"=w1129:string[])  [unwired: 10 in]
            n573 = Index Array(array=w1120, index #1=14 ("index"), index #2=15 ("index")) -> (element #1=w1125:string, element #2=w1121:string)
            n574 = Number To Decimal String(number="Ageing Gas") -> (decimal integer string=w1133:string)  [unwired: 1 in]
            n575 = Number To Decimal String(number=w1134) -> (decimal integer string=w1132:string)  [unwired: 1 in]
            n576 = Decimal String To Number(string=w1121, default (0L)=w1123) -> (number=w1122:dbl)  [unwired: 1 in, 1 out]
            n577 = Decimal String To Number(string=w1125, default (0L)=w1123) -> (number=w1124:dbl)  [unwired: 1 in, 1 out]
            n578 = property on="Inlet temp Age" class="DigNum (strict)"("Value"=w1124) -> ()  [unwired: 2 in, 2 out]
            n579 = property on="Flow rate Age" class="DigNum (strict)"("Value"=w1122) -> ()  [unwired: 2 in, 2 out]
            n580 = Build Array (concatenate)(w1133, w1132, w1129) -> (w1128:string[])
            n581 = shared-variable "NI-cRIO9074-018C1D8D\\Library 1.lvlib\\Ageing Variables"(w1128) -> ()  [unwired: 1 in, 1 out]
          }
        }
        "Test Compiled" <- w1114
      }
      frame "convert to num" {
        n582 = local read "EditPos Subc"() -> (w1143:T3)
        n583 = Unbundle By Name(w1143) -> ("Row"=w1144:i32, "Column"=w1141:i32)
        n584 = Equal?(x=w1141, y=7) -> (x = y?=w1140:bool)
        n585 = case shown="False" w1140 {
          tunnel: w1144 -> [_ w1149]
          tunnel: w1141 -> [_ w1147]
          tunnel: w1143 -> [_ _]
          frame True {
          }
          frame False {
            n586 = local read "Sub-Cycle Pattern"() -> (w1146:string[][])
            n587 = call "Conv to num.vi"("Column"=w1147, "Row"=w1149, "Array"=w1146) -> ("result string"=w1148:string)  [unwired: 8 in]
            n588 = Replace Array Subset(array=w1146, new element=w1148, index (row)=w1149, index (col)=w1147) -> (w1145:string[][])
            n589 = local write "Sub-Cycle Pattern"(w1145) -> ()
          }
        }
      }
      frame "check scycle name" {
        n590 = local read "Sub-Cycle Name"() -> (w1150:T5)
        n591 = call <vilib>:"Search and Replace Pattern.vi"("string"=w1150, "regular expression (\"\")"="[^0-9a-zA-Z ]" ("format string"), "replace string (\"\")"="", "replace all? (F)"=TRUE) -> ("result string"=w1156:string)  [unwired: 1 in, 1 out]
        n592 = Not Equal?(x=w1156, y=w1150) -> (x != y?=w1155:bool)
        n593 = case shown="False" w1155 {
          tunnel: w1156 -> [w1157 w1158]
          tunnel: [w1157 w1158] -> w1151
          frame False {
          }
          frame True {
            n594 = One Button Dialog(message="Unsuitable character for the file name!") -> ()  [unwired: 1 in, 1 out]
          }
        }
        n595 = local write "Sub-Cycle Name"(w1151) -> ()
      }
      frame "check cycle name" {
        n596 = local read "Cycle Name"() -> (w1160:T5)
        n597 = call <vilib>:"Search and Replace Pattern.vi"("string"=w1160, "regular expression (\"\")"="[^0-9a-zA-Z ]" ("format string"), "replace string (\"\")"="", "replace all? (F)"=TRUE) -> ("result string"=w1166:string)  [unwired: 1 in, 1 out]
        n598 = Not Equal?(x=w1166, y=w1160) -> (x != y?=w1165:bool)
        n599 = case shown="False" w1165 {
          tunnel: w1166 -> [w1167 w1168]
          tunnel: [w1167 w1168] -> w1161
          frame False {
          }
          frame True {
            n600 = One Button Dialog(message="Unsuitable character for the file name!") -> ()  [unwired: 1 in, 1 out]
          }
        }
        n601 = local write "Cycle Name"(w1161) -> ()
      }
      frame "Multigas connect" {
        n602 = flat-sequence {
          frame #0 {
            "Connected?" <- TRUE
          }
        }
      }
      frame "Multigas disconnect" {
      }
    }
    n603 = local read "stop 2"() -> (w556:bool)
  }
  n604 = disable-structure shown="Disabled" {
    frame Disabled {
      n605 = while {
        tunnel: [w1209] -> w1194
        tunnel: [w1208] -> w1193
        stop <- w1205 stop-if-true
        n606 = TCP Open Connection(address="192.168.1.3", remote port or service name=u16 7700) -> (connection ID=w1209:refnum<k5>, error out=w1208:errorcluster)  [unwired: 3 in]
        n607 = Unbundle By Name(w1208) -> ("status"=w1210:bool)
        n608 = Not(x=w1210) -> (.not. x?=w1206:bool)
        n609 = Or(x=w1206, y="stop TCP") -> (x .or. y?=w1205:bool)
      }
      n610 = Concatenate Strings("\r", "\n") -> (w1182:string)
      n611 = Concatenate Strings("MSSM,0,1,1" ("data in"), w1182) -> (w1189:string)
      n612 = TCP Write(connection ID=w1194, data in=w1189, error in (no error)=w1193) -> (connection ID out=w1197:refnum<k5>, error out=w1198:errorcluster)  [unwired: 1 in, 1 out]
      n613 = Concatenate Strings("MSMD,1,7,1,1,1,1,2,1,1,3,1,1,4,1,1,5,1,1,6,1,1,7,1" ("data in"), w1182) -> (w1184:string)
      n614 = TCP Write(connection ID=w1197, data in=w1184, error in (no error)=w1198) -> (connection ID out=w1195:refnum<k5>, error out=w1196:errorcluster)  [unwired: 1 in, 1 out]
      n615 = Concatenate Strings("MSTT,1,0" ("string"), w1182) -> (w1183:string)
      n616 = TCP Write(connection ID=w1195, data in=w1183, error in (no error)=w1196) -> (connection ID out=w1181:refnum<k5>, error out=w1180:errorcluster)  [unwired: 1 in, 1 out]
      n617 = UDP Open(9:500 ("timeout ms (25000)"), 11:u16 7701 ("port")) -> ()  [unwired: 3 in, 3 out]
      n618 = UDP Read(timeout ms (25000)=500) -> (data out=w1172:string)  [unwired: 3 in, 4 out]
      n619 = while {
        shift-right: [w1201] -> _
        shift-left: w1172 -> [w1204]
        tunnel: [w1202] -> w1173 mode=indexing
        stop <- w1199 stop-if-true
        n620 = Search/Split String(string=w1204, search string/char (-)=",") -> (substring before match=w1202:string, match + rest of string=w1201:string)  [unwired: 1 in, 1 out]
        n621 = String Length(string=w1201) -> (length=w1200:i32)
        n622 = Equal To 0?(x=w1200) -> (x = 0?=w1199:bool)
      }
      n623 = call "7170string to array.vi"("Array in"=w1173) -> ()  [unwired: 4 in, 1 out]
      n624 = UDP Close() -> ()  [unwired: 2 in, 2 out]
      n625 = Concatenate Strings("MSTP,0,0" ("string"), "\r", "\n") -> (w1176:string)
      n626 = TCP Write(data in=w1176) -> (connection ID out=w1178:refnum<k5>, error out=w1179:errorcluster)  [unwired: 3 in, 1 out]
      n627 = TCP Close Connection(connection ID=w1178, error in (no error)=w1179) -> ()  [unwired: 1 in, 2 out]
    }
    frame Enabled {
    }
  }
  n628 = local write "stop 2"(w9) -> ()
  n629 = node-c288(w6) -> ()  [unwired: 1 out]
  "Table" <- string[][] [] ("Table")
